vi "DebugProg.vi"() -> ()   [LabVIEW 2012]
uses:
  Instance           5 17Saved   DebugProg .vi
panel:
  out "output array 3":u8[](array[numeric])
  out "VOC Port and states":string[][](array[string])
  out "VOC INPUT PORT states":bool[](array[boolean])
  out "Output Alg Ports":bool[](array[boolean])
  out "Sizes":i32[](array[numeric])
  out "output array 2":u8[](array[numeric])
  out "ALG INPUT PORT states":bool[](array[boolean])
  out "ALG Port and states":string[][](array[string])
  out "Input Alg Ports":bool[](array[boolean])
  out "Output ALG Msg Last Iter":string[][](table)=[["CODE", "PARAM"]]
  out "Output VOC Msg Last Iter":string[][](table)=[["CODE", "PARAM"]]
  out "Curr step ALG msg counter":i32
  out "Curr step VOC MSG counter":i32
  out "Params":string[](array[string])
  in  "STEP SIZE":i32(knob)=1 scale=1.0..10.0
  in  "Mode":bool
  in  "stop 2":bool
  in  "run":bool
  out "Result Input FOR VOC":u8[](array[numeric])
  out "output array":cluster{i32, "Value":string, i32}[](array[cluster])
  in  "Numeric":u8
  in  "Tab Control":T1(tab)=enum."Input VOC Ports "
  out "ALG MSG queue":u8(slide) scale=0.0..5.0
  in  "send msg":bool
  in  "ALG MSG  PARAM":string
  in  "ALG MSG TYPE":string(combo)="0"
  in  "ALG MSG  CODE":string(combo)="1"
  out "VOC MSG queue":u8(slide) scale=0.0..5.0
  in  "send voc msg 2":bool
  in  "VOC MSG  PARAM":string
  in  "VOC MSG TYPE":string(combo)="0"
  in  "VOC MSG  CODE":string(combo)
  in  "New value\n(ALG ports)":i8 min=0
  in  "Controlable\n(ALG ports)":bool
  in  "Set new value\n(ALG ports)":bool
  in  "ALG Input Ports":i32(listbox)
  in  "New value (VOC ports)":i8 min=0
  in  "Controlable (VOC ports)":bool
  in  "Set new value (VOC ports)":bool
  in  "VOC Input Ports":i32(listbox)
  in  "ALG Param type":string(combo)
  in  "ALG Last Interation MSG":i32(listbox)
  out "Alg States":string[][](table)
  out "Output Alg Msg":string[][](table)=[["CODE", "PARAM"]]
  in  "VOC Last Interation MSG":i32(listbox)
  in  "VOC Param type":string(combo)
  out "Output VOC Msg LOG":string[][](table)=[["CODE", "PARAM"]]
  out "VOC States":string[][](table)
  in  "Save as new test":bool
  in  "Save changes in current test":bool
  in  "TEST":string="script_port: 8 /*index*/, 0 /* СЦЕНАРИЙ_ЛОГ_ВХОД_ПИТ_ВЕНТИЛЯТОРА*/ \r\nscript_port: 9 /*index*/, 0 /* СЦЕНАРИЙ_ЛОГ_ВХОД_ПИТ_РЕГ_Т*/ \r\nscript_port: 10 /*index*/, 0 /* СЦЕНАРИЙ_ЛОГ_ВХОД_НАС_ОХЛ*/ \r\nscript_port: 11 /*index*/, 0 /* СЦЕНАРИЙ_ЛОГ_ВХОД_ВАК_НАСОСА*/ \r\nscript_port: 12 /*index*/, 0 /* СЦЕНАРИЙ_ЛОГ_ВХОД_ЗАТВОР_ВАК*/ \r\nscript_port: 13 /*index*/, 0 /* СЦЕНАРИЙ_ЛОГ_ВХОД_САПУН*/ \r\nscript_port: 14 /*index*/, 0 /* СЦЕНАРИЙ_ЛОГ_ВХОД_УСТР_ПЛАВ_ПУСКА*/ \r\nscript_port: 15 /*index*/, 0 /* СЦЕНАРИЙ_ЛОГ_ВХОД_РЕГ_УР*/ \r\nscript_port: 16 /*index*/, 0 /* СЦЕНАРИЙ_ЛОГ_ВХОД_КОМПРЕССОР*/ \r\n\n\n\n\n\n\n\n"
  in  "Tests List":i32(listbox)
  out "voc code":i32[](array[numeric])=[-1, -1, -1, -1, -1, -1, -1, -1, -1, -1, -1, -1, -1, -1, -1, -1, -1, -1, -1, -1, -1, -1, -1, -1, -1, -1, -1, -1, -1, -1, -1, -1, -1, -1, -1, -1, -1, -1, -1, -1, -1, -1, -1, -1, -1, -1, -1, -1, -1, -1, -1, -1, -1, -1, -1, -1, -1, -1, -1, -1, -1, -1, -1, -1, -1, -1, -1, -1, -1, -1, -1, -1, -1, -1, -1, -1, -1, -1, -1, -1, -1, -1, -1, -1, -1, -1, -1, -1, -1, -1, -1, -1, -1, -1, -1, -1, -1, -1, -1, -1, -1, -1, -1, -1, -1, -1, -1, -1, -1, -1, -1, -1, -1, -1, -1, -1, -1, -1, -1, -1, -1, -1, -1, -1, -1, -1, -1, -1, -1, -1, -1, -1, -1, -1, -1, -1, -1, -1, -1, -1, -1, -1, -1, -1, -1, -1, -1, -1, -1, -1, -1, -1, -1, -1, -1, -1, -1, -1, -1, -1, -1, -1, -1, -1, -1, -1, -1, -1, -1, -1, -1, -1, -1, -1, -1, -1, -1, -1, -1, -1, -1, -1, -1, -1, -1, -1, -1, -1, -1, -1, -1, -1, -1, -1, -1, -1, -1, -1, -1, -1, -1, -1, -1, -1, -1, -1, -1, -1, -1, -1, -1, -1, -1, -1, -1, -1, -1, -1, -1, -1, -1, -1, -1, -1, -1, -1, -1, -1, -1, -1, -1, -1, -1, -1, -1, -1, -1, -1, -1, -1, -1, -1, -1, -1, -1, -1, -1, -1, -1, -1]
  out "VOC Out MSG Codes":string[](array[string])=["4", "5", "6", "7", "8", "9", "10", "11", "12", "13", "14", "15", "16", "17", "18", "19", "20", "21", "22", "23", "24", "25", "26", "27", "28", "29", "30", "31", "32", "33"]
  out "VOC Out MSG Names":string[](array[string])=["ПК_ТЕСТ_ГУИ_ОШИБКА_КОДА_КОМАНДЫ_ОТ_ГУИ", "ПК_ТЕСТ_ГУИ_ТЕМПЕРАТУРА_ВОДЫ_В_БАКЕ_ИЗМЕНИЛАСЬ", "ПК_ТЕСТ_ГУИ_ТЕМПЕРАТУРА_ВОДЫ_В_РУБАШКЕ_ИЗМЕНИЛАСЬ", "ПК_ТЕСТ_ГУИ_ТЕМПЕРАТУРА_НАСОСА_ИЗМЕНИЛАСЬ", "ПК_ТЕСТ_ГУИ_ВОДА_В_БАКЕ_ЗАКИПЕЛА", "ПК_ТЕСТ_ГУИ_ВОДА_В_БАКЕ_ЗАМЕРЗЛА", "ПК_ТЕСТ_ГУИ_ТЕМПЕРАТУРА_ВОДЫ_В_БАКЕ_СЛИШКОМ_ВЫСОКАЯ", "ПК_ТЕСТ_ГУИ_ТЕМПЕРАТУРА_ВОДЫ_В_БАКЕ_СЛИШКОМ_НИЗКАЯ", "ПК_ТЕСТ_ГУИ_ТЕМПЕРАТУРА_ОКУЖАЮЩЕЙ_СРЕДЫ_ИЗМЕНИЛАСЬ", "ПК_ТЕСТ_ГУИ_ТЕМПЕРАТУРА_ОКУЖАЮЩЕЙ_СРЕДЫ_СЛИШКОМ_ВЫСОКАЯ", "ПК_ТЕСТ_ГУИ_ТЕМПЕРАТУРА_ОКУЖАЮЩЕЙ_СРЕДЫ_СЛИШКОМ_НИЗКАЯ", "ПК_ТЕСТ_ГУИ_УРОВЕНЬ_ВОДЫ_НОРМ", "ПК_ТЕСТ_ГУИ_УРОВЕНЬ_ВОДЫ_MAX", "ПК_ТЕСТ_ГУИ_УРОВЕНЬ_ВОДЫ_MIN", "ПК_ТЕСТ_ГУИ_ДАВЛЕНИЕ_В_ТРУБЕ_СИДЕРОСТАТА_ИЗМЕНИЛОСЬ", "ПК_ТЕСТ_ГУИ_ДАВЛЕНИЕ_В_ТРУБЕ_СЛИШКОМ_ВЫСОКОЕ", "ПК_ТЕСТ_ГУИ_ДАВЛЕНИЕ_В_ТРУБЕ_СЛИШКОМ_НИЗКОЕ", "ПК_ТЕСТ_ГУИ_ДАВЛЕНИЕ_В_ПАТРУБКЕ_ИЗМЕНИЛОСЬ", "ПК_ТЕСТ_ГУИ_ДАВЛЕНИЕ_В_ПАТРУБКЕ_СЛИШКОМ_ВЫСОКОЕ", "ПК_ТЕСТ_ГУИ_ДАВЛЕНИЕ_В_ПАТРУБКЕ_СЛИШКОМ_НИЗКОЕ", "ПК_ТЕСТ_ГУИ_ДАВЛЕНИЕ_В_БАКЕ_КОМПРЕССОРА_ИЗМЕНИЛОСЬ", "ПК_ТЕСТ_ГУИ_ДАВЛЕНИЕ_В_КОМПРЕССОРЕ_СЛИШКОМ_НИЗКОЕ", "ПК_ТЕСТ_ГУИ_ОШИБКА_ПОПЫТКА_ОТКРЫТЬ_САПУН_ПРИ_ОТКРЫТОМ_ЗАТВОРЕ", "ПК_ТЕСТ_ГУИ_ОШИБКА_ПОПЫТКА_ОТКРЫТЬ_ЗАТВОР_ПРИ_ОТКРЫТОМ_САПУНЕ", "ПК_ТЕСТ_ГУИ_ОШИБКА_ДАВЛЕНИЕ_ПАТРУБКА_ВЫШЕ_ДАВЛЕНИЯ_ТРУБЫ", "ПК_ТЕСТ_ГУИ_ОШИБКА_ВКЛЮЧЕНИЕ_НАГРЕВА_ПРИ_НИЗКОМ_УРОВНЕ_ВОДЫ", "ПК_ТЕСТ_ГУИ_ПОПЫТКА_ЗАПУСКА_УСТР_ПЛАВ_ПУСКА_БЕЗ_ПИТАНИЯ", "ПК_ТЕСТ_ГУИ_ОШИБКА_ВКЛЮЧЕНИЕ_НАСОСА_ОХЛ_ПРИ_НИЗКОМ_УРОВНЕ_ВОДЫ", "ПК_ТЕСТ_ГУИ_ОШИБКА_ПЕРЕГРЕВ_ВАК_НАСОСА", "ПК_ТЕСТ_ГУИ_ОШИБКА_ОТКЛЮЧЕНИЕ_ПИТАНИЯ_ВКН_ПРИ_ЗАПУЩЕННОМ_ВКН"]
  out "output VOC array":cluster{i32, "Value":string, i32}[](array[cluster])=[{-1, "Value"="", 0}, {-1, "Value"="", 0}, {-1, "Value"="", 0}, {-1, "Value"="", 0}, {-1, "Value"="", 0}, {-1, "Value"="", 0}, {-1, "Value"="", 0}, {-1, "Value"="", 0}, {-1, "Value"="", 0}, {-1, "Value"="", 0}, {-1, "Value"="", 0}, {-1, "Value"="", 0}, {-1, "Value"="", 0}, {-1, "Value"="", 0}, {-1, "Value"="", 0}]
  out "input VOC array":cluster{i32, "Value":string, i32}[](array[cluster])
  out "AY states array":cluster{u32, u8}[](array[cluster])
  out "ALG output array":cluster{i32, "Value":string, i32}[](array[cluster])=[{-1, "Value"="", 0}, {-1, "Value"="", 0}, {-1, "Value"="", 0}, {-1, "Value"="", 0}, {-1, "Value"="", 0}]
  out "voc states array":cluster{u32, u8}[](array[cluster])
  out "ALG input array":cluster{i32, "Value":string, i32}[](array[cluster])
  out "VOC_STATES_SET":string[][](array[string])=[["Начало", " ", " ", " ", " ", " "], ["Начало", "НекорректноеСобытие", " ", " ", " ", " "], ["Начало", " ", " ", " ", " ", " "], ["Останов", " ", " ", " ", " ", " "], ["Начало", "Неисправность_вентилятора", " ", " ", " ", " "], ["Включение", "Вентилятор_ВКЛЮЧЕН", " ", " ", " ", " "], ["Выключение", "Вентилятор_ВЫКЛЮЧЕН", " ", " ", " ", " "], ["Начало", "Неисправность_Регулятора_Температуры", " ", " ", " ", " "], ["Включение", "Контроль_температуры_ВКЛЮЧЕН", "Временное_Отключение", "Кипение", " ", " "], ["Включение", "Контроль_температуры_ВЫКЛЮЧЕН", "СамопроизвольноеОхлаждение", "СамопроивольныйНагрев", "Замерзло", "ТепловоеРавновесие"], ["Начало", "Неисправность_регулятора_уровня", " ", " ", " ", " "], ["Включение", "Контроль_Рег_Уровня_ВКЛЮЧЕН", " ", " ", " ", " "], ["Включение", "Контроль_Рег_Уровня_ВЫКЛЮЧЕН", " ", " ", " ", " "], ["Начало", "Неисправность_Насоса_Охлаждения", " ", " ", " ", " "], ["Включение", "Контроль_Насоса_Охлажд_ВКЛЮЧЕН", "НАГРЕВ_НАСОСА_ОХЛАЖД_ВОДЫ", "ОХЛАЖД_НАСОСА_НАГРЕВ_ВОДЫ", "ТепловоеРавновесие", "Авария"], ["Включение", "Контроль_Насоса_Охлажд_ВЫКЛЮЧЕН", "САМОПРОИЗВ_ОХЛАЖД_НАСОСА", "САМОПРОИЗВ_НАГРЕВ_НАСОСА", "ТепловоеРавновесие", " "], ["Начало", "Неисправность_Сапуна", " ", " ", " ", " "], ["Открытие", "Сапун_ОТКРЫТ", " ", " ", " ", " "], ["Выключение", "Сапун_ЗАКРЫТ", " ", " ", " ", " "], ["Начало", "Неисправность_Затвора", " ", " ", " ", " "], ["Открытие", "Затвор_ОТКРЫТ", " ", " ", " ", " "], ["Закрытие", "Затвор_ЗАКРЫТ", " ", " ", " ", " "], ["Начало", "Неисправность_питания_насоса", " ", " ", " ", " "], ["Включение", "Питание_ПОДАНО", " ", " ", " ", " "], ["Выключение", "Задержка_перед_отключением", "Питание_ОТКЛЮЧЕНО", " ", " ", " "], ["Начало", "Неисправность_устр_плав_пуска", " ", " ", " ", " "], ["Включение", "Устр_Плав_Пуска_ЗАПУЩЕНО", "Вакуум", " ", " ", " "], ["Выключение", "Устр_Плав_Пуска_ОСТАНОВЛЕНО", " ", " ", " ", " "], ["Начало", "Исправность_Компрессора", "Неисправность_Компрессора", " ", " ", " "]]
  out "VOC_PROC":string[](array[string])=["Инициализация", "ЧтениеКольцевогоБуфера", "ЗАПОЛНЕНИЕ_ДОСТОВЕРНОСТЕЙ", "АварийноеЗавершениеРаботы", "УПРАВЛЕНИЕ_ВЕНТИЛЯТОРОМ", "ВКЛЮЧЕНИЕ_ВЕНТИЛЯТОРА", "ВЫКЛЮЧЕНИЕ_ВЕНТИЛЯТОРА", "УПРАВЛЕНИЕ_ТЕМПЕРАТУРОЙ", "ВКЛЮЧЕНИЕ_РЕГ_ТЕМПЕРАТУРЫ", "ВЫКЛЮЧЕНИЕ_РЕГ_ТЕМПЕРАТУРЫ", "УПРАВЛЕНИЕ_РЕГУЛЯТОРОМ_УР_ВОДЫ_В_БАКЕ", "ВКЛЮЧЕНИЕ_РЕГ_УРОВНЯ", "ВЫКЛЮЧЕНИЕ_РЕГ_УРОВНЯ", "УПРАВЛЕНИЕ_НАСОСОМ_ОХЛАЖДЕНИЯ", "ВКЛЮЧЕНИЕ_НАСОСА_ОХЛАЖД", "ВЫКЛЮЧЕНИЕ_НАСОСА_ОХЛАЖД", "УПРАВЛЕНИЕ_САПУНОМ", "ОТКРЫТИЕ_САПУНА", "ЗАКРЫТИЕ_САПУНА", "УПРАВЛЕНИЕ_ЗАТВОРОМ", "ОТКРЫТИЕ_ЗАТВОРА", "ЗАКРЫТИЕ_ЗАТВОРА", "УПРАВЛЕНИЕ_ПИТАНИЕМ_ВКН", "ПОДАЧА_ПИТАНИЯ_НА_ВКН", "ОТКЛЮЧЕНИЕ_ПИТАНИЯ_ВКН", "УПРАВЛЕНИЕ_УСТР_ПЛАВ_ПУСКА", "ЗАПУСК_УСТР_ПЛАВ_ПУСКА", "ОСТАНОВ_УСТР_ПЛАВ_ПУСКА", "УПРАВЛЕНИЕ_КОМПРЕССОРОМ"]
  out "Alg Out MSG Codes":string[](array[string])=["0", "1", "2", "3", "4", "5", "6", "7", "8", "9", "10", "11", "12", "13", "14", "15", "16", "41", "42", "43", "44", "45", "46", "47", "48", "49", "50", "51", "52", "53", "54", "55", "56", "57", "58", "59", "60", "61", "62", "63", "64", "65", "66", "67", "68", "69", "70", "71", "72", "73", "74", "75", "76", "77", "78", "79", "80", "81", "82", "83", "84", "85", "86", "87", "88", "89", "90", "91", "92", "93", "94", "95", "96", "97", "98", "99", "100", "101", "102", "103", "104", "105", "106", "107", "108", "109", "110", "111", "112", "113", "114", "115", "116", "117", "118", "119", "120", "121", "122", "123", "124", "125", "126", "127", "128", "129", "130", "135"]
  out "Alg Out MSG Names":string[](array[string])=["ПК_ГУИ_УРОВЕНЬ_ВОДЫ_В_БАКЕ_ОХЛАЖДЕНИЯ_НИЗКИЙ", "ПК_ГУИ_УРОВЕНЬ_ВОДЫ_В_БАКЕ_ОХЛАЖДЕНИЯ_ВЫСОКИЙ", "ПК_ГУИ_УРОВЕНЬ_ВОДЫ_В_БАКЕ_ОХЛАЖДЕНИЯ_В_НОРМЕ", "ПК_ГУИ_ОТКАЗ_ДАТЧИКОВ_УРОВНЯ", "ПК_ГУИ_ТЕМПЕРАТУРА_ВОДЫ_В_БАКЕ_ОХЛАЖДЕНИЯ_НИЗКАЯ", "ПК_ГУИ_ТЕМПЕРАТУРА_ВОДЫ_В_БАКЕ_ОХЛАЖДЕНИЯ_ВЫСОКАЯ", "ПК_ГУИ_ТЕМПЕРАТУРА_ВОДЫ_В_БАКЕ_ОХЛАЖДЕНИЯ_В_НОРМЕ", "ПК_ГУИ_ТЕМПЕРАТУРА_ВОДЫ_В_РУБАШКЕ_ОХЛАЖДЕНИЯ_НИЗКАЯ", "ПК_ГУИ_ТЕМПЕРАТУРА_ВОДЫ_В_РУБАШКЕ_ОХЛАЖДЕНИЯ_ВЫСОКАЯ", "ПК_ГУИ_ТЕМПЕРАТУРА_ВОДЫ_В_РУБАШКЕ_ОХЛАЖДЕНИЯ_В_НОРМЕ", "ПК_ГУИ_ДАВЛЕНИЕ_В_ВАКУУМНОЙ_ТРУБЕ_В_НОРМЕ", "ПК_ГУИ_ДАВЛЕНИЕ_В_ВАКУУМНОЙ_ТРУБЕ_ВНЕ_НОРМЫ", "ПК_ГУИ_СКОРОСТЬ_ОТКАЧКИ_В_НОРМЕ", "ПК_ГУИ_СКОРОСТЬ_ОТКАЧКИ_НИЖЕ_НОРМЫ", "ПК_ГУИ_ДАВЛЕНИЕ_В_БАКЕ_КОМПРЕССОРА_В_НОРМЕ", "ПК_ГУИ_ДАВЛЕНИЕ_В_БАКЕ_КОМПРЕССОРА_ВЫШЕ_НОРМЫ", "ПК_ГУИ_ДАВЛЕНИЕ_В_БАКЕ_КОМПРЕССОРА_НИЖЕ_НОРМЫ", "ПК_ГУИ_ОТКАЗ_ОТКРЫТИЯ_ЗАТВОРА_ВАКУУМНОГО", "ПК_ГУИ_ОТКАЗ_ЗАКРЫТИЯ_ЗАТВОРА_ВАКУУМНОГО", "ПК_ГУИ_ОТКАЗ_ОТКРЫТИЯ_САПУНА", "ПК_ГУИ_ОТКАЗ_ЗАКРЫТИЯ_САПУНА", "ПК_ГУИ_ОТКАЗ_ВКЛЮЧЕНИЯ_ВЕНТИЛЯТОРА", "ПК_ГУИ_ОТКАЗ_ВЫКЛЮЧЕНИЯ_ВЕНТИЛЯТОРА", "ПК_ГУИ_ОТКАЗ_ВКЛЮЧЕНИЯ_УСТР_ПЛАВ_ПУСКА", "ПК_ГУИ_ОТКАЗ_ВЫКЛЮЧЕНИЯ_УСТР_ПЛАВ_ПУСКА", "ПК_ГУИ_ОТКАЗ_ВКЛЮЧЕНИЯ_РЕГУЛЯТОРА_ТЕМПЕРАТУРЫ", "ПК_ГУИ_ОТКАЗ_ВЫКЛЮЧЕНИЯ_РЕГУЛЯТОРА_ТЕМПЕРАТУРЫ", "ПК_ГУИ_ОТКАЗ_ВКЛЮЧЕНИЯ_РЕГУЛЯТОРА_УРОВНЯ", "ПК_ГУИ_ОТКАЗ_ВЫКЛЮЧЕНИЯ_РЕГУЛЯТОРА_УРОВНЯ", "ПК_ГУИ_ОТКАЗ_ВКЛЮЧЕНИЯ_НАСОСА_ОХЛАЖДЕНИЯ", "ПК_ГУИ_ОТКАЗ_ВЫКЛЮЧЕНИЯ_НАСОСА_ОХЛАЖДЕНИЯ", "ПК_ГУИ_ИДЕТ_ВАКУУМИРОВАНИЕ_ОТКАЗ_ВЫПОЛНЕНИЯ_КОМАНДЫ", "ПК_ГУИ_НЕТ_УСЛОВИЙ_ДЛЯ_ВЫПОЛНЕНИЯ_КОМАНДЫ", "ПК_ГУИ_УРОВЕНЬ_ВОДЫ_В_БАКЕ_ОХЛАЖДЕНИЯ_ВНЕ_НОРМЫ_ОТКАЗ_ВЫПОЛНЕНИ", "ПК_ГУИ_ОТРИЦАТЕЛЬНАЯ_ТЕМПЕРАТУРА_ВОДЫ_ОТКАЗ_ВЫПОЛНЕНИЯ_КОМАНДЫ", "ПК_ГУИ_ДАВЛЕНИЕ_В_ПАТРУБКЕ_НЕ_УМЕНЬШАЕТСЯ", "ПК_ГУИ_ДАВЛЕНИЕ_В_ВАК_ТРУБЕ_НЕ_УМЕНЬШАЕТСЯ", "ПК_ГУИ_ВАКУУМИРОВАНИЕ_УСПЕШНО_ЗАВЕРШЕНО", "ПК_ГУИ_ОТКАЗ_ВКЛЮЧЕНИЯ_ПИТАНИЯ_ВАКУУМНОГО_НАСОСА", "ПК_ГУИ_ОТКАЗ_ВЫКЛЮЧЕНИЯ_ПИТАНИЯ_ВАКУУМНОГО_НАСОСА", "ПК_ГУИ_АВАРИЯ_НЕДОСТОВЕРНЫЕ_ДАННЫЕ_ОБОРУДОВАНИЯ_ВАК_СИСТЕМЫ", "ПК_ГУИ_ВЕНТИЛЯТОР_ВКЛЮЧЕН", "ПК_ГУИ_ВЕНТИЛЯТОР_ВЫКЛЮЧЕН", "ПК_ГУИ_СПОНТАННОЕ_ВЫКЛЮЧЕНИЕ_ВЕНТИЛЯТОРА", "ПК_ГУИ_СПОНТАННОЕ_ВКЛЮЧЕНИЕ_ВЕНТИЛЯТОРА", "ПК_ГУИ_ЗАТВОР_ВАКУУМНЫЙ_ОТКРЫТ", "ПК_ГУИ_ЗАТВОР_ВАКУУМНЫЙ_ЗАКРЫТ", "ПК_ГУИ_СРЕДНЕЕ_СОСТОЯНИЕ_ЗАТВОРА_ВАКУУМНОГО", "ПК_ГУИ_СОСТОЯНИЕ_ОШИБКИ_ЗАТВОРА_ВАКУУМНОГО", "ПК_ГУИ_СПОНТАННОЕ_ОТКРЫТИЕ_ЗАТ_ВАКУУМНОГО", "ПК_ГУИ_СПОНТАННОЕ_ЗАКРЫТИЕ_ЗАТ_ВАКУУМНОГО", "ПК_ГУИ_САПУН_ОТКРЫТ", "ПК_ГУИ_САПУН_ЗАКРЫТ", "ПК_ГУИ_СПОНТАННОЕ_ОТКРЫТИЕ_САПУНА", "ПК_ГУИ_СПОНТАННОЕ_ЗАКРЫТИЕ_САПУНА", "ПК_ГУИ_ПИТАНИЕ_ВАКУУМНОГО_НАСОСА_ВКЛЮЧЕНО", "ПК_ГУИ_ПИТАНИЕ_ВАКУУМНОГО_НАСОСА_ВЫКЛЮЧЕНО", "ПК_ГУИ_СПОНТАННОЕ_ВКЛЮЧЕНИЕ_ВАКУУМНОГО_НАСОСА", "ПК_ГУИ_СПОНТАННОЕ_ВЫКЛЮЧЕНИЕ_ВАКУУМНОГО_НАСОСА", "ПК_ГУИ_ПИТАНИЕ_РЕГУЛЯТОРА_ТЕМПЕРАТУРЫ_ВКЛЮЧЕНО", "ПК_ГУИ_ПИТАНИЕ_РЕГУЛЯТОРА_ТЕМПЕРАТУРЫ_ВЫКЛЮЧЕНО", "ПК_ГУИ_СПОНТАННОЕ_ВКЛЮЧЕНИЕ_РЕГУЛЯТОРА_ТЕМПЕРАТУРЫ", "ПК_ГУИ_СПОНТАННОЕ_ВЫКЛЮЧЕНИЕ_РЕГУЛЯТОРА_ТЕМПЕРАТУРЫ", "ПК_ГУИ_ПИТАНИЕ_РЕГУЛЯТОРА_УРОВНЯ_ВКЛЮЧЕНО", "ПК_ГУИ_ПИТАНИЕ_РЕГУЛЯТОРА_УРОВНЯ_ВЫКЛЮЧЕНО", "ПК_ГУИ_СПОНТАННОЕ_ВКЛЮЧЕНИЕ_РЕГУЛЯТОРА_УРОВНЯ", "ПК_ГУИ_СПОНТАННОЕ_ВЫКЛЮЧЕНИЕ_РЕГУЛЯТОРА_УРОВНЯ", "ПК_ГУИ_ПИТАНИЕ_НАСОСА_ОХЛАЖДЕНИЯ_ВКЛЮЧЕНО", "ПК_ГУИ_ПИТАНИЕ_НАСОСА_ОХЛАЖДЕНИЯ_ВЫКЛЮЧЕНО", "ПК_ГУИ_СПОНТАННОЕ_ВКЛЮЧЕНИЕ_НАСОСА_ОХЛАЖДЕНИЯ", "ПК_ГУИ_СПОНТАННОЕ_ВЫКЛЮЧЕНИЕ_НАСОСА_ОХЛАЖДЕНИЯ", "ПК_ГУИ_УСТРОЙСТВО_ПЛАВНОГО_ПУСКА_ВКЛЮЧЕНО", "ПК_ГУИ_УСТРОЙСТВО_ПЛАВНОГО_ПУСКА_ВЫКЛЮЧЕНО", "ПК_ГУИ_СПОНТАННОЕ_ВКЛЮЧЕНИЕ_УСТРОЙСТВА_ПЛАВНОГО_ПУСКА", "ПК_ГУИ_СПОНТАННОЕ_ВЫКЛЮЧЕНИЕ_УСТРОЙСТВА_ПЛАВНОГО_ПУСКА", "ПК_ГУИ_ОТКАЗ_ВАКУУМИРОВАНИЯ", "ПК_ГУИ_ОТКАЗ_ВКЛЮЧЕНИЯ_ВАКУУМНОЙ_ПОДСИСТЕМЫ", "ПК_ГУИ_ОТКАЗ_ВЫКЛЮЧЕНИЯ_ВАКУУМНОЙ_ПОДСИСТЕМЫ", "ПК_ГУИ_ЕСТЬ_ДОСТОВЕРНОСТЬ_КОНТРОЛЯ_ОТКРЫТИЯ_ЗАТВОРА_ВАКУУМНОГО", "ПК_ГУИ_НЕТ_ДОСТОВЕРНОСТИ_КОНТРОЛЯ_ОТКРЫТИЯ_ЗАТВОРА_ВАКУУМНОГО", "ПК_ГУИ_ЕСТЬ_ДОСТОВЕРНОСТЬ_КОНТРОЛЯ_ЗАКРЫТИЯ_ЗАТВОРА_ВАКУУМНОГО", "ПК_ГУИ_НЕТ_ДОСТОВЕРНОСТИ_КОНТРОЛЯ_ЗАКРЫТИЯ_ЗАТВОРА_ВАКУУМНОГО", "ПК_ГУИ_ЕСТЬ_ДОСТОВЕРНОСТЬ_КОНТРОЛЯ_САПУНА", "ПК_ГУИ_НЕТ_ДОСТОВЕРНОСТИ_КОНТРОЛЯ_САПУНА", "ПК_ГУИ_ЕСТЬ_ДОСТОВЕРНОСТЬ_КОНТРОЛЯ_УСТР_ПЛАВ_ПУСКА", "ПК_ГУИ_НЕТ_ДОСТОВЕРНОСТИ_КОНТРОЛЯ_УСТР_ПЛАВ_ПУСКА", "ПК_ГУИ_ЕСТЬ_ДОСТОВЕРНОСТЬ_КОНТРОЛЯ_ПИТ_ВАК_НАСОСА", "ПК_ГУИ_НЕТ_ДОСТОВЕРНОСТИ_КОНТРОЛЯ_ПИТ_ВАК_НАСОСА", "ПК_ГУИ_ЕСТЬ_ДОСТОВЕРНОСТЬ_КОНТРОЛЯ_ПИТ_ВЕНТИЛЯТОРА", "ПК_ГУИ_НЕТ_ДОСТОВЕРНОСТИ_КОНТРОЛЯ_ПИТ_ВЕНТИЛЯТОРА", "ПК_ГУИ_ЕСТЬ_ДОСТОВЕРНОСТЬ_РЕГ_ТЕМПЕРАТУРЫ", "ПК_ГУИ_НЕТ_ДОСТОВЕРНОСТИ_КОНТРОЛЯ_ПИТ_РЕГ_ТЕМПЕРАТУРЫ", "ПК_ГУИ_ЕСТЬ_ДОСТОВЕРНОСТЬ_РЕГ_УРОВНЯ", "ПК_ГУИ_НЕТ_ДОСТОВЕРНОСТИ_КОНТРОЛЯ_ПИТ_РЕГ_УРОВНЯ", "ПК_ГУИ_ЕСТЬ_ДОСТОВЕРНОСТЬ_МИНИМ_УР_ВОДЫ", "ПК_ГУИ_НЕТ_ДОСТОВЕРНОСТИ_МИНИМ_УР_ВОДЫ", "ПК_ГУИ_ЕСТЬ_ДОСТОВЕРНОСТЬ_МАКСИМ_УР_ВОДЫ", "ПК_ГУИ_НЕТ_ДОСТОВЕРНОСТИ_МАКСИМ_УР_ВОДЫ", "ПК_ГУИ_ЕСТЬ_ДОСТОВЕРНОСТЬ_КОНТРОЛЯ_ПИТ_НАСОСА_ОХЛ", "ПК_ГУИ_НЕТ_ДОСТОВЕРНОСТИ_КОНТРОЛЯ_ПИТ_НАСОСА_ОХЛ", "ПК_ГУИ_ВАКУУМИРОВАНИЕ_ТРУБЫ_ВКЛЮЧЕНО", "ПК_ГУИ_ВАКУУМИРОВАНИЕ_ТРУБЫ_ВЫКЛЮЧЕНО", "ПК_ГУИ_ФП_P_ВбакеКомпрессора", "ПК_ГУИ_ФП_P_Впатрубке", "ПК_ГУИ_ФП_T_Врубашке", "ПК_ГУИ_ФП_T_Вбаке", "ПК_ГУИ_ФП_P_ВтрубеСидер", "ПК_ГУИ_ОШИБКА_КОДА_КОМАНДЫ_ОТ_ГУИ"]
  out "AY_STATES_SET":string[][](array[string])=[["Начало", "ВосстановлениеУправления", "НачалоРаботы", " ", " ", " ", " ", " ", " ", " ", " ", " ", " ", " ", " ", " ", " ", " ", " ", " ", " ", " ", " ", " ", " ", " ", " ", " ", " ", " "], ["Начало", " ", " ", " ", " ", " ", " ", " ", " ", " ", " ", " ", " ", " ", " ", " ", " ", " ", " ", " ", " ", " ", " ", " ", " ", " ", " ", " ", " ", " "], ["Начало", "ОстановПроцессов", "СообК_ГУИ_НЕТ_ДОСТОВЕРНОСТИ", "НарушениеСвязи", " ", " ", " ", " ", " ", " ", " ", " ", " ", " ", " ", " ", " ", " ", " ", " ", " ", " ", " ", " ", " ", " ", " ", " ", " ", " "], ["Начало", "СменаСостоянияВКЛ", "СменаСостоянияВЫКЛ", "ТрафикПауза", "НарушениеСвязи", " ", " ", " ", " ", " ", " ", " ", " ", " ", " ", " ", " ", " ", " ", " ", " ", " ", " ", " ", " ", " ", " ", " ", " ", " "], ["Начало", "СообК_ГУИ_ЕСТЬ_ДОСТОВЕРНОСТЬ", "ОжиданиеНедостоверности", "СообК_ГУИ_НЕТ_ДОСТОВЕРНОСТИ", "ОжиданиеЕстьДостоверность", "НарушениеСвязи", " ", " ", " ", " ", " ", " ", " ", " ", " ", " ", " ", " ", " ", " ", " ", " ", " ", " ", " ", " ", " ", " ", " ", " "], ["Начало", "СообК_ГУИ_ЕСТЬ_ДОСТОВЕРНОСТЬ", "ОжиданиеНедостоверности", "СообК_ГУИ_НЕТ_ДОСТОВЕРНОСТИ", "ОжиданиеЕстьДостоверность", "НарушениеСвязи", " ", " ", " ", " ", " ", " ", " ", " ", " ", " ", " ", " ", " ", " ", " ", " ", " ", " ", " ", " ", " ", " ", " ", " "], ["Начало", "СообК_ГУИ_ЕСТЬ_ДОСТОВЕРНОСТЬ", "ОжиданиеНедостоверности", "СообК_ГУИ_НЕТ_ДОСТОВЕРНОСТИ", "ОжиданиеЕстьДостоверность", "НарушениеСвязи", " ", " ", " ", " ", " ", " ", " ", " ", " ", " ", " ", " ", " ", " ", " ", " ", " ", " ", " ", " ", " ", " ", " ", " "], ["Начало", "СообК_ГУИ_ЕСТЬ_ДОСТОВЕРНОСТЬ", "ОжиданиеНедостоверности", "СообК_ГУИ_НЕТ_ДОСТОВЕРНОСТИ", "ОжиданиеЕстьДостоверность", "НарушениеСвязи", " ", " ", " ", " ", " ", " ", " ", " ", " ", " ", " ", " ", " ", " ", " ", " ", " ", " ", " ", " ", " ", " ", " ", " "], ["Начало", "СообК_ГУИ_ЕСТЬ_ДОСТОВЕРНОСТЬ", "ОжиданиеНедостоверности", "СообК_ГУИ_НЕТ_ДОСТОВЕРНОСТИ", "ОжиданиеЕстьДостоверность", "НарушениеСвязи", " ", " ", " ", " ", " ", " ", " ", " ", " ", " ", " ", " ", " ", " ", " ", " ", " ", " ", " ", " ", " ", " ", " ", " "], ["Начало", "СообК_ГУИ_ЕСТЬ_ДОСТОВЕРНОСТЬ", "ОжиданиеНедостоверности", "СообК_ГУИ_НЕТ_ДОСТОВЕРНОСТИ", "ОжиданиеЕстьДостоверность", "НарушениеСвязи", " ", " ", " ", " ", " ", " ", " ", " ", " ", " ", " ", " ", " ", " ", " ", " ", " ", " ", " ", " ", " ", " ", " ", " "], ["Начало", "СообК_ГУИ_ЕСТЬ_ДОСТОВЕРНОСТЬ", "ОжиданиеНедостоверности", "СообК_ГУИ_НЕТ_ДОСТОВЕРНОСТИ", "ОжиданиеЕстьДостоверность", "НарушениеСвязи", " ", " ", " ", " ", " ", " ", " ", " ", " ", " ", " ", " ", " ", " ", " ", " ", " ", " ", " ", " ", " ", " ", " ", " "], ["Начало", "СообК_ГУИ_ЕСТЬ_ДОСТОВЕРНОСТЬ", "ОжиданиеНедостоверности", "СообК_ГУИ_НЕТ_ДОСТОВЕРНОСТИ", "ОжиданиеЕстьДостоверность", "НарушениеСвязи", " ", " ", " ", " ", " ", " ", " ", " ", " ", " ", " ", " ", " ", " ", " ", " ", " ", " ", " ", " ", " ", " ", " ", " "], ["Начало", "СообК_ГУИ_ЕСТЬ_ДОСТОВЕРНОСТЬ", "ОжиданиеНедостоверности", "СообК_ГУИ_НЕТ_ДОСТОВЕРНОСТИ", "ОжиданиеЕстьДостоверность", "НарушениеСвязи", " ", " ", " ", " ", " ", " ", " ", " ", " ", " ", " ", " ", " ", " ", " ", " ", " ", " ", " ", " ", " ", " ", " ", " "], ["Начало", "СообК_ГУИ_ЕСТЬ_ДОСТОВЕРНОСТЬ", "ОжиданиеНедостоверности", "СообК_ГУИ_НЕТ_ДОСТОВЕРНОСТИ", "ОжиданиеЕстьДостоверность", "НарушениеСвязи", " ", " ", " ", " ", " ", " ", " ", " ", " ", " ", " ", " ", " ", " ", " ", " ", " ", " ", " ", " ", " ", " ", " ", " "], ["Начало", "СообК_ГУИ_ЕСТЬ_ДОСТОВЕРНОСТЬ", "ОжиданиеНедостоверности", "СообК_ГУИ_НЕТ_ДОСТОВЕРНОСТИ", "ОжиданиеЕстьДостоверность", "НарушениеСвязи", " ", " ", " ", " ", " ", " ", " ", " ", " ", " ", " ", " ", " ", " ", " ", " ", " ", " ", " ", " ", " ", " ", " ", " "], ["Начало", " ", " ", " ", " ", " ", " ", " ", " ", " ", " ", " ", " ", " ", " ", " ", " ", " ", " ", " ", " ", " ", " ", " ", " ", " ", " ", " ", " ", " "], ["Начало", " ", " ", " ", " ", " ", " ", " ", " ", " ", " ", " ", " ", " ", " ", " ", " ", " ", " ", " ", " ", " ", " ", " ", " ", " ", " ", " ", " ", " "], ["Начало", "КонтрольВыполненияК", "КонтрольИзмененияНП", "НекорректноеСобытие", "НарушениеСвязи", " ", " ", " ", " ", " ", " ", " ", " ", " ", " ", " ", " ", " ", " ", " ", " ", " ", " ", " ", " ", " ", " ", " ", " ", " "], ["Анализ", "ПодтверждениеИзмененияНП", "НекорректноеСобытие", "НарушениеСвязи", " ", " ", " ", " ", " ", " ", " ", " ", " ", " ", " ", " ", " ", " ", " ", " ", " ", " ", " ", " ", " ", " ", " ", " ", " ", " "], ["Анализ", "НекорректноеСобытие", "ПередачаСообщенияСПараметромГУИ", "НарушениеСвязи", " ", " ", " ", " ", " ", " ", " ", " ", " ", " ", " ", " ", " ", " ", " ", " ", " ", " ", " ", " ", " ", " ", " ", " ", " ", " "], ["Начало", "КонтрольИзменения", "СообщОбИзменении", "ТрафикПауза", "НарушениеСвязи", " ", " ", " ", " ", " ", " ", " ", " ", " ", " ", " ", " ", " ", " ", " ", " ", " ", " ", " ", " ", " ", " ", " ", " ", " "], ["Начало", "КонтрольИзменения", "СообщОбИзменении", "ТрафикПауза", "НарушениеСвязи", " ", " ", " ", " ", " ", " ", " ", " ", " ", " ", " ", " ", " ", " ", " ", " ", " ", " ", " ", " ", " ", " ", " ", " ", " "], ["Начало", "КонтрольИзменения", "СообщОбИзменении", "ТрафикПауза", "НарушениеСвязи", " ", " ", " ", " ", " ", " ", " ", " ", " ", " ", " ", " ", " ", " ", " ", " ", " ", " ", " ", " ", " ", " ", " ", " ", " "], ["Начало", "КонтрольИзменения", "СообщОбИзменении", "ТрафикПауза", "НарушениеСвязи", " ", " ", " ", " ", " ", " ", " ", " ", " ", " ", " ", " ", " ", " ", " ", " ", " ", " ", " ", " ", " ", " ", " ", " ", " "], ["Начало", "КонтрольИзменения", "СообщОбИзменении", "ТрафикПауза", "НарушениеСвязи", " ", " ", " ", " ", " ", " ", " ", " ", " ", " ", " ", " ", " ", " ", " ", " ", " ", " ", " ", " ", " ", " ", " ", " ", " "], ["Начало", "АнализОткачки", " ", " ", " ", " ", " ", " ", " ", " ", " ", " ", " ", " ", " ", " ", " ", " ", " ", " ", " ", " ", " ", " ", " ", " ", " ", " ", " ", " "], ["Начало", "ДавлениеНормальное", "ДавлениеВысокое", "Задержка", "НарушениеСвязи", " ", " ", " ", " ", " ", " ", " ", " ", " ", " ", " ", " ", " ", " ", " ", " ", " ", " ", " ", " ", " ", " ", " ", " ", " "], ["Начало", "НизкийУровеньВоды", "ВысокийУровеньВоды", "УровеньВодыВнорме", "Задержка", "НарушениеСвязи", " ", " ", " ", " ", " ", " ", " ", " ", " ", " ", " ", " ", " ", " ", " ", " ", " ", " ", " ", " ", " ", " ", " ", " "], ["Начало", "НизкаяТемператураВоды", "ВысокаяТемператураВоды", "ТемператураВнорме", "Задержка", "НарушениеСвязи", " ", " ", " ", " ", " ", " ", " ", " ", " ", " ", " ", " ", " ", " ", " ", " ", " ", " ", " ", " ", " ", " ", " ", " "], ["Начало", "НизкаяТемператураВоды", "ВысокаяТемператураВоды", "ТемператураВнорме", "Задержка", "НарушениеСвязи", " ", " ", " ", " ", " ", " ", " ", " ", " ", " ", " ", " ", " ", " ", " ", " ", " ", " ", " ", " ", " ", " ", " ", " "], ["Начало", "НизкоеДавление", "ДавлениеВнорме", "Задержка", "НарушениеСвязи", " ", " ", " ", " ", " ", " ", " ", " ", " ", " ", " ", " ", " ", " ", " ", " ", " ", " ", " ", " ", " ", " ", " ", " ", " "], ["Начало", "КонтрольВключения", "ПередачаСообщения", "Ошибка", "НарушениеСвязи", " ", " ", " ", " ", " ", " ", " ", " ", " ", " ", " ", " ", " ", " ", " ", " ", " ", " ", " ", " ", " ", " ", " ", " ", " "], ["Начало", "КонтрольВыключения", "ПередачаСообщения", "Ошибка", "НарушениеСвязи", " ", " ", " ", " ", " ", " ", " ", " ", " ", " ", " ", " ", " ", " ", " ", " ", " ", " ", " ", " ", " ", " ", " ", " ", " "], ["Начало", "СменаСостоянияВКЛ", "СменаСостоянияВЫКЛ", "НарушениеСвязи", " ", " ", " ", " ", " ", " ", " ", " ", " ", " ", " ", " ", " ", " ", " ", " ", " ", " ", " ", " ", " ", " ", " ", " ", " ", " "], ["Контроль", "Ошибка", "НарушениеСвязи", " ", " ", " ", " ", " ", " ", " ", " ", " ", " ", " ", " ", " ", " ", " ", " ", " ", " ", " ", " ", " ", " ", " ", " ", " ", " ", " "], ["Контроль", "Ошибка", "НарушениеСвязи", " ", " ", " ", " ", " ", " ", " ", " ", " ", " ", " ", " ", " ", " ", " ", " ", " ", " ", " ", " ", " ", " ", " ", " ", " ", " ", " "], ["Начало", "СменаСостоянияСреднего", "СменаСостоянияЗакрытия", "СменаСостоянияОткрытия", "СменаСостоянияОшибки", "НарушениеСвязи", " ", " ", " ", " ", " ", " ", " ", " ", " ", " ", " ", " ", " ", " ", " ", " ", " ", " ", " ", " ", " ", " ", " ", " "], ["Начало", "Контроль", "ПередачаСообщения", "Ошибка", "НарушениеСвязи", " ", " ", " ", " ", " ", " ", " ", " ", " ", " ", " ", " ", " ", " ", " ", " ", " ", " ", " ", " ", " ", " ", " ", " ", " "], ["Начало", "Контроль", "ПередачаСообщения", "Ошибка", "НарушениеСвязи", " ", " ", " ", " ", " ", " ", " ", " ", " ", " ", " ", " ", " ", " ", " ", " ", " ", " ", " ", " ", " ", " ", " ", " ", " "], ["КонтрольЗакрытия", "Ошибка", "НарушениеСвязи", " ", " ", " ", " ", " ", " ", " ", " ", " ", " ", " ", " ", " ", " ", " ", " ", " ", " ", " ", " ", " ", " ", " ", " ", " ", " ", " "], ["Контроль", "Ошибка", "НарушениеСвязи", " ", " ", " ", " ", " ", " ", " ", " ", " ", " ", " ", " ", " ", " ", " ", " ", " ", " ", " ", " ", " ", " ", " ", " ", " ", " ", " "], ["Начало", "КонтрольОткрытия", "ПередачаСообщения", "Ошибка", "НарушениеСвязи", " ", " ", " ", " ", " ", " ", " ", " ", " ", " ", " ", " ", " ", " ", " ", " ", " ", " ", " ", " ", " ", " ", " ", " ", " "], ["Начало", "КонтрольЗакрытия", "ПередачаСообщения", "Ошибка", "НарушениеСвязи", " ", " ", " ", " ", " ", " ", " ", " ", " ", " ", " ", " ", " ", " ", " ", " ", " ", " ", " ", " ", " ", " ", " ", " ", " "], ["Начало", "СменаСостоянияВКЛ", "СменаСостоянияВЫКЛ", "НарушениеСвязи", " ", " ", " ", " ", " ", " ", " ", " ", " ", " ", " ", " ", " ", " ", " ", " ", " ", " ", " ", " ", " ", " ", " ", " ", " ", " "], ["КонтрольЗакрытия", "Ошибка", "НарушениеСвязи", " ", " ", " ", " ", " ", " ", " ", " ", " ", " ", " ", " ", " ", " ", " ", " ", " ", " ", " ", " ", " ", " ", " ", " ", " ", " ", " "], ["Контроль", "Ошибка", "НарушениеСвязи", " ", " ", " ", " ", " ", " ", " ", " ", " ", " ", " ", " ", " ", " ", " ", " ", " ", " ", " ", " ", " ", " ", " ", " ", " ", " ", " "], ["Начало", "КонтрольВключения", "ПередачаСообщения", "Ошибка", "НарушениеСвязи", " ", " ", " ", " ", " ", " ", " ", " ", " ", " ", " ", " ", " ", " ", " ", " ", " ", " ", " ", " ", " ", " ", " ", " ", " "], ["Начало", "КонтрольВыключения", "Ошибка", "НарушениеСвязи", "ПередачаСообщения", " ", " ", " ", " ", " ", " ", " ", " ", " ", " ", " ", " ", " ", " ", " ", " ", " ", " ", " ", " ", " ", " ", " ", " ", " "], ["Начало", "СменаСостоянияВКЛ", "СменаСостоянияВЫКЛ", "НарушениеСвязи", " ", " ", " ", " ", " ", " ", " ", " ", " ", " ", " ", " ", " ", " ", " ", " ", " ", " ", " ", " ", " ", " ", " ", " ", " ", " "], ["Контроль", "Ошибка", "НарушениеСвязи", " ", " ", " ", " ", " ", " ", " ", " ", " ", " ", " ", " ", " ", " ", " ", " ", " ", " ", " ", " ", " ", " ", " ", " ", " ", " ", " "], ["Контроль", "Ошибка", "НарушениеСвязи", " ", " ", " ", " ", " ", " ", " ", " ", " ", " ", " ", " ", " ", " ", " ", " ", " ", " ", " ", " ", " ", " ", " ", " ", " ", " ", " "], ["Начало", "КонтрольВключения", "ПередачаСообщения", "Ошибка", "НарушениеСвязи", " ", " ", " ", " ", " ", " ", " ", " ", " ", " ", " ", " ", " ", " ", " ", " ", " ", " ", " ", " ", " ", " ", " ", " ", " "], ["Начало", "КонтрольВыключения", "ПередачаСообщения", "Ошибка", "НарушениеСвязи", " ", " ", " ", " ", " ", " ", " ", " ", " ", " ", " ", " ", " ", " ", " ", " ", " ", " ", " ", " ", " ", " ", " ", " ", " "], ["Начало", "СменаСостоянияВКЛ", "СменаСостоянияВЫКЛ", "НарушениеСвязи", " ", " ", " ", " ", " ", " ", " ", " ", " ", " ", " ", " ", " ", " ", " ", " ", " ", " ", " ", " ", " ", " ", " ", " ", " ", " "], ["Контроль", "Ошибка", "НарушениеСвязи", " ", " ", " ", " ", " ", " ", " ", " ", " ", " ", " ", " ", " ", " ", " ", " ", " ", " ", " ", " ", " ", " ", " ", " ", " ", " ", " "], ["Контроль", "Ошибка", "НарушениеСвязи", " ", " ", " ", " ", " ", " ", " ", " ", " ", " ", " ", " ", " ", " ", " ", " ", " ", " ", " ", " ", " ", " ", " ", " ", " ", " ", " "], ["Начало", "Контроль", "ПередачаСообщения", "Ошибка", "НарушениеСвязи", " ", " ", " ", " ", " ", " ", " ", " ", " ", " ", " ", " ", " ", " ", " ", " ", " ", " ", " ", " ", " ", " ", " ", " ", " "], ["Начало", "Контроль", "ПередачаСообщения", "Ошибка", "НарушениеСвязи", " ", " ", " ", " ", " ", " ", " ", " ", " ", " ", " ", " ", " ", " ", " ", " ", " ", " ", " ", " ", " ", " ", " ", " ", " "], ["Начало", "СменаСостоянияВКЛ", "СменаСостоянияВЫКЛ", "НарушениеСвязи", " ", " ", " ", " ", " ", " ", " ", " ", " ", " ", " ", " ", " ", " ", " ", " ", " ", " ", " ", " ", " ", " ", " ", " ", " ", " "], ["Контроль", "Ошибка", "НарушениеСвязи", " ", " ", " ", " ", " ", " ", " ", " ", " ", " ", " ", " ", " ", " ", " ", " ", " ", " ", " ", " ", " ", " ", " ", " ", " ", " ", " "], ["Контроль", "Ошибка", "НарушениеСвязи", " ", " ", " ", " ", " ", " ", " ", " ", " ", " ", " ", " ", " ", " ", " ", " ", " ", " ", " ", " ", " ", " ", " ", " ", " ", " ", " "], ["Начало", "ВключениеПитания", "Контроль", "ПередачаСообщения", "Ошибка", "НарушениеСвязи", " ", " ", " ", " ", " ", " ", " ", " ", " ", " ", " ", " ", " ", " ", " ", " ", " ", " ", " ", " ", " ", " ", " ", " "], ["Начало", "Контроль", "ПередачаСообщения", "Ошибка", "НарушениеСвязи", " ", " ", " ", " ", " ", " ", " ", " ", " ", " ", " ", " ", " ", " ", " ", " ", " ", " ", " ", " ", " ", " ", " ", " ", " "], ["Начало", "СменаСостоянияВКЛ", "СменаСостоянияВЫКЛ", "НарушениеСвязи", " ", " ", " ", " ", " ", " ", " ", " ", " ", " ", " ", " ", " ", " ", " ", " ", " ", " ", " ", " ", " ", " ", " ", " ", " ", " "], ["Контроль", "Ошибка", "НарушениеСвязи", " ", " ", " ", " ", " ", " ", " ", " ", " ", " ", " ", " ", " ", " ", " ", " ", " ", " ", " ", " ", " ", " ", " ", " ", " ", " ", " "], ["Контроль", "Ошибка", "НарушениеСвязи", " ", " ", " ", " ", " ", " ", " ", " ", " ", " ", " ", " ", " ", " ", " ", " ", " ", " ", " ", " ", " ", " ", " ", " ", " ", " ", " "], ["Начало", "Контроль", "ПередачаСообщения", "Ошибка", "НарушениеСвязи", " ", " ", " ", " ", " ", " ", " ", " ", " ", " ", " ", " ", " ", " ", " ", " ", " ", " ", " ", " ", " ", " ", " ", " ", " "], ["Начало", "КонтрольВыключения", "ПередачаСообщения", "Ошибка", "НарушениеСвязи", " ", " ", " ", " ", " ", " ", " ", " ", " ", " ", " ", " ", " ", " ", " ", " ", " ", " ", " ", " ", " ", " ", " ", " ", " "], ["Начало", "СменаСостоянияВКЛ", "СменаСостоянияВЫКЛ", "НарушениеСвязи", " ", " ", " ", " ", " ", " ", " ", " ", " ", " ", " ", " ", " ", " ", " ", " ", " ", " ", " ", " ", " ", " ", " ", " ", " ", " "], ["Контроль", "Ошибка", "НарушениеСвязи", " ", " ", " ", " ", " ", " ", " ", " ", " ", " ", " ", " ", " ", " ", " ", " ", " ", " ", " ", " ", " ", " ", " ", " ", " ", " ", " "], ["Контроль", "Ошибка", "НарушениеСвязи", " ", " ", " ", " ", " ", " ", " ", " ", " ", " ", " ", " ", " ", " ", " ", " ", " ", " ", " ", " ", " ", " ", " ", " ", " ", " ", " "], ["Начало", "ПроверкаНеобходимостиВакуумирования", "ПередачаСообщения", "КонтрольВключенияВакПодсистемы", "ЗапоминаемДавлениеВвакуумнойТрубе", "КонтрольТемпературыРубашки", "КонтрольРаботыОборудования", "КонтрольДавления", "СообщениеОКонцеВакуумирования", "ПаузаНаРазвакуумированиеТрубы", "ПаузаНаОткачкуВвакуумнойТрубе", "ПроверкаУменьшенияДавленияВпатрубке", "ОткачкаОтсутствует", "ВыключениеВакуумнойПодсистемы", "СообщениеОбОтказеВакуумирования", "НарушениеСвязи", " ", " ", " ", " ", " ", " ", " ", " ", " ", " ", " ", " ", " ", " "], ["Начало", "ПередачаСообщения", "ВыключениеВакуумнойПодсистемы", "НарушениеСвязи", " ", " ", " ", " ", " ", " ", " ", " ", " ", " ", " ", " ", " ", " ", " ", " ", " ", " ", " ", " ", " ", " ", " ", " ", " ", " "], ["Начало", "ВключениеПитанияРегУровня", "КонтрольВключенияПитРегУр", "КонтрольГотовностиУровняВодыБО", "ВключениеРегТ", "КонтрольВключенияРегТ", "КонтрольПревышенияТемпературыВодыБО", "КонтрольГотовностиТемпературыВодыБО", "ВключаемВентилятор", "КонтрольВключенияВентилятора", "КонтрольВключенияПитанияНасосаОхлаждения", "КонтрольЗакрытияЗатвораВакуумного", "КонтрольОткрытияСапуна", "КонтрольТемпературыРубашки", "ПодачаПитанияНаВакуумныйНасос", "КонтрольПитанияВакуумногоНасоса", "ВключениеУстройстваПлавногоПуска", "КонтрольВлюченияПлавногоПуска", "ТаймаутПередЗакрытиемСапуна", "ЗакрытиеСапуна", "КонтрольЗакрытияСапуна", "ЗапоминаемДавлениеВпатрубке", "КонтрольДавления", "ПаузаНаОткачкуВпатрубке", "ПроверкаУменьшенияДавленияВпатрубке", "КонтрольОткрытияЗВ", "Ошибка", "ВыключениеПоОшибке", "СообщениеОбОтказеВакуумирования", "НарушениеСвязи"], ["Начало", "КонтрольЗакрытияЗатвораВакуумного", "КонтрольОткрытияСапуна", "ТаймаутПередВыключениемПитанияВакуумногоНасоса", "ВыключаемУППВакуумногоНасоса", "КонтрольВыключенияПитанияУППВакуумногоНасоса", "КонтрольВыключенияПитанияВакуумногоНасоса", "КонтрольВыключенияНасосаОхлаждения", "КонтрольВыключенияВентилятора", "СообщениеОбОтказеВыклВакСистемы", "НарушениеСвязи", " ", " ", " ", " ", " ", " ", " ", " ", " ", " ", " ", " ", " ", " ", " ", " ", " ", " ", " "]]
  out "AY_PROC":string[](array[string])=["Инициализация", "ОстановВсехПроцессовИстартПроцИнициализация", "КонтрольДостоверности", "КонтрольДостоверностиОткрытияЗатвораВакуумного", "КонтрольДостоверностиОткрЗатВакуумного", "КонтрольДостоверностиЗакрЗатВакуумного", "КонтрольДостоверностиСостоянияСапуна", "КонтрольДостоверностиСостоянияУстройстваПлавПуска", "КонтрольДостоверностиСостоянияПитанияВакуумногоНасоса", "КонтрольДостоверностиСостоянияПитанияВентилятора", "КонтрольДостоверностиСостоянияПитанияРегТемпературы", "КонтрольДостоверностиСостоянияПитанияРегУровня", "КонтрольДостоверностиУровняВодыМинимум", "КонтрольДостоверностиУровняВодыМаксимум", "КонтрольДостоверностиСостоянияПитанияНасОхлаждения", "ЧтениеФактПараметров_с_Датчиков", "РЕГУЛЯТОР_ТРАФИКА", "ЧтениеКольцевогоБуфера", "ОбработкаКомандИзмененияНП_от_ГУИ", "ОбработкаКомандУправления_от_ГУИ", "КонтрольИзменения_ФП_P_ВбакеКомпрессора", "КонтрольИзменения_ФП_P_Впатрубке", "КонтрольИзменения_ФП_T_Врубашке", "КонтрольИзменения_ФП_T_Вбаке", "КонтрольИзменения_ФП_P_ВтрубеСидер", "КонтрольВеличиныОткачкиВауумнойТрубыСидеростата", "КонтрольГотовностиВакуума_в_Вакуумной_Трубе", "КонтрольУровняВодыБакаОхлаждения", "КонтрольТемпературыВодыБакаОхлаждения", "КонтрольТемпературыРубашкиОхлаждения", "КонтрольДавленияВбакеКомпрессора", "ВКЛ_ПИТ_ВЕНТИЛЯТОР", "ВЫК_ПИТ_ВЕНТИЛЯТОР", "КонтрольСостоянияПитанияВентилятора", "КонтрольСпонтанногоВыключенияВентилятора", "КонтрольСпонтанногоВключенияВентилятора", "КонтрольСостоянияЗатвораВакуумного", "ОТКР_ЗАТВОР_ВАК", "ЗАКР_ЗАТВОР_ВАК", "КонтрольСпонтанногоЗакрытияЗатвораВакуумного", "КонтрольСпонтанногоОткрытияЗатвораВакуумного", "ОТКР_САПУН", "ЗАКР_САПУН", "КонтрольСостоянияПитанияСапуна", "КонтрольСпонтанногоЗакрытияСапуна", "КонтрольСпонтанногоОткрытияСапуна", "ВКЛ_ПИТ_ВАК_НАСОСА", "ВЫК_ПИТ_ВАК_НАСОСА", "КонтрольСостоянияПитанияВакуумногоНасоса", "КонтрольСпонтанногоВыключенияВакНасоса", "КонтрольСпонтанногоВключенияВакНасоса", "ВКЛ_ПИТ_РЕГ_Т", "ВЫК_ПИТ_РЕГ_Т", "КонтрольСостоянияПитанияРЕГ_Т", "КонтрольСпонтанногоВыключенияРЕГ_Т", "КонтрольСпонтанногоВключенияРЕГ_Т", "ВКЛ_ПИТ_РЕГ_УР", "ВЫК_ПИТ_РЕГ_УР", "КонтрольСостоянияПитанияРЕГ_УР", "КонтрольСпонтанногоВыключенияРЕГ_УР", "КонтрольСпонтанногоВключенияРЕГ_УР", "ВКЛ_ПИТ_НАС_ОХЛ", "ВЫК_ПИТ_НАС_ОХЛ", "КонтрольСостоянияПитанияНАС_ОХЛ", "КонтрольСпонтанногоВыключенияНасосаОхлаждения", "КонтрольСпонтанногоВключенияНасосаОхлаждения", "ВКЛ_УСТР_ПЛАВ_ПУСКА", "ВЫК_УСТР_ПЛАВ_ПУСКА", "КонтрольСостоянияПитанияПЛАВ_ПУСКА", "КонтрольСпонтанногоВыключенияПлавнПуска", "КонтрольСпонтанногоВключенияПлавнПуска", "ВКЛ_ВАКУУМИРОВАНИЕ_ТРУБЫ", "ВЫК_ВАКУУМИРОВАНИЕ_ТРУБЫ", "ВКЛ_ВАКУУМНУЮ_ПОДСИСТЕМУ", "ВЫК_ВАКУУМНУЮ_ПОДСИСТЕМУ"]
  out "Init  VOC INPUT":u8[](array[numeric])
  out "Alg Input":i32[](array[numeric])=[2, 2, 2, 2, 2, 2, 2, 2, 2, 2, 2]
  out "Init ALG input":u8[](array[numeric])
  in  "stop":bool
  # "К_ОТКР_ЗАТВОР_ВАК"
  # "К_ЗАКР_ЗАТВОР_ВАК"
  # "У_ПИТ_ВЕНТИЛЯТОРА"
  # "К_САПУН"
  # "У_ПИТ_РЕГ_Т"
  # "К_УСТР_ПЛАВ_ПУСКА"
  # "У_ПИТ_НАС_ОХЛ"
  # "К_ПИТ_ВАК_НАСОСА"
  # "У_ПИТ_ВАК_НАСОСА"
  # "К_ВЕНТИЛЯТОР"
  # "У_ЗАТВОР_ВАК"
  # "К_ПИТ_РЕГ_Т"
  # "У_САПУН"
  # "К_ПИТ_РЕГ_УР"
  # "У_УСТР_ПЛАВ_ПУСКА"
  # "К_УР_ВОДЫ_MIN"
  # "У_ПИТ_РЕГ_УР"
  # "К_УР_ВОДЫ_MAX"
  # "К_ПИТ_НАСОС_ОХЛ"
  # "К_ЛОГ_ВХОД_P_ВбакеКомпрессора"
  # "К_ЛОГ_ВХОД_P_Впатрубке"
  # "К_ЛОГ_ВХОД_T_Врубашке"
  # "К_ЛОГ_ВХОД_T_Вбаке"
  # "К_ЛОГ_ВХОД_P_ВтрубеСидер"
  # "STEP MODE"
  # "CONTINUOUS MODE"
  # "ALG MSG Generation"
  # "VOC MSG Generation"
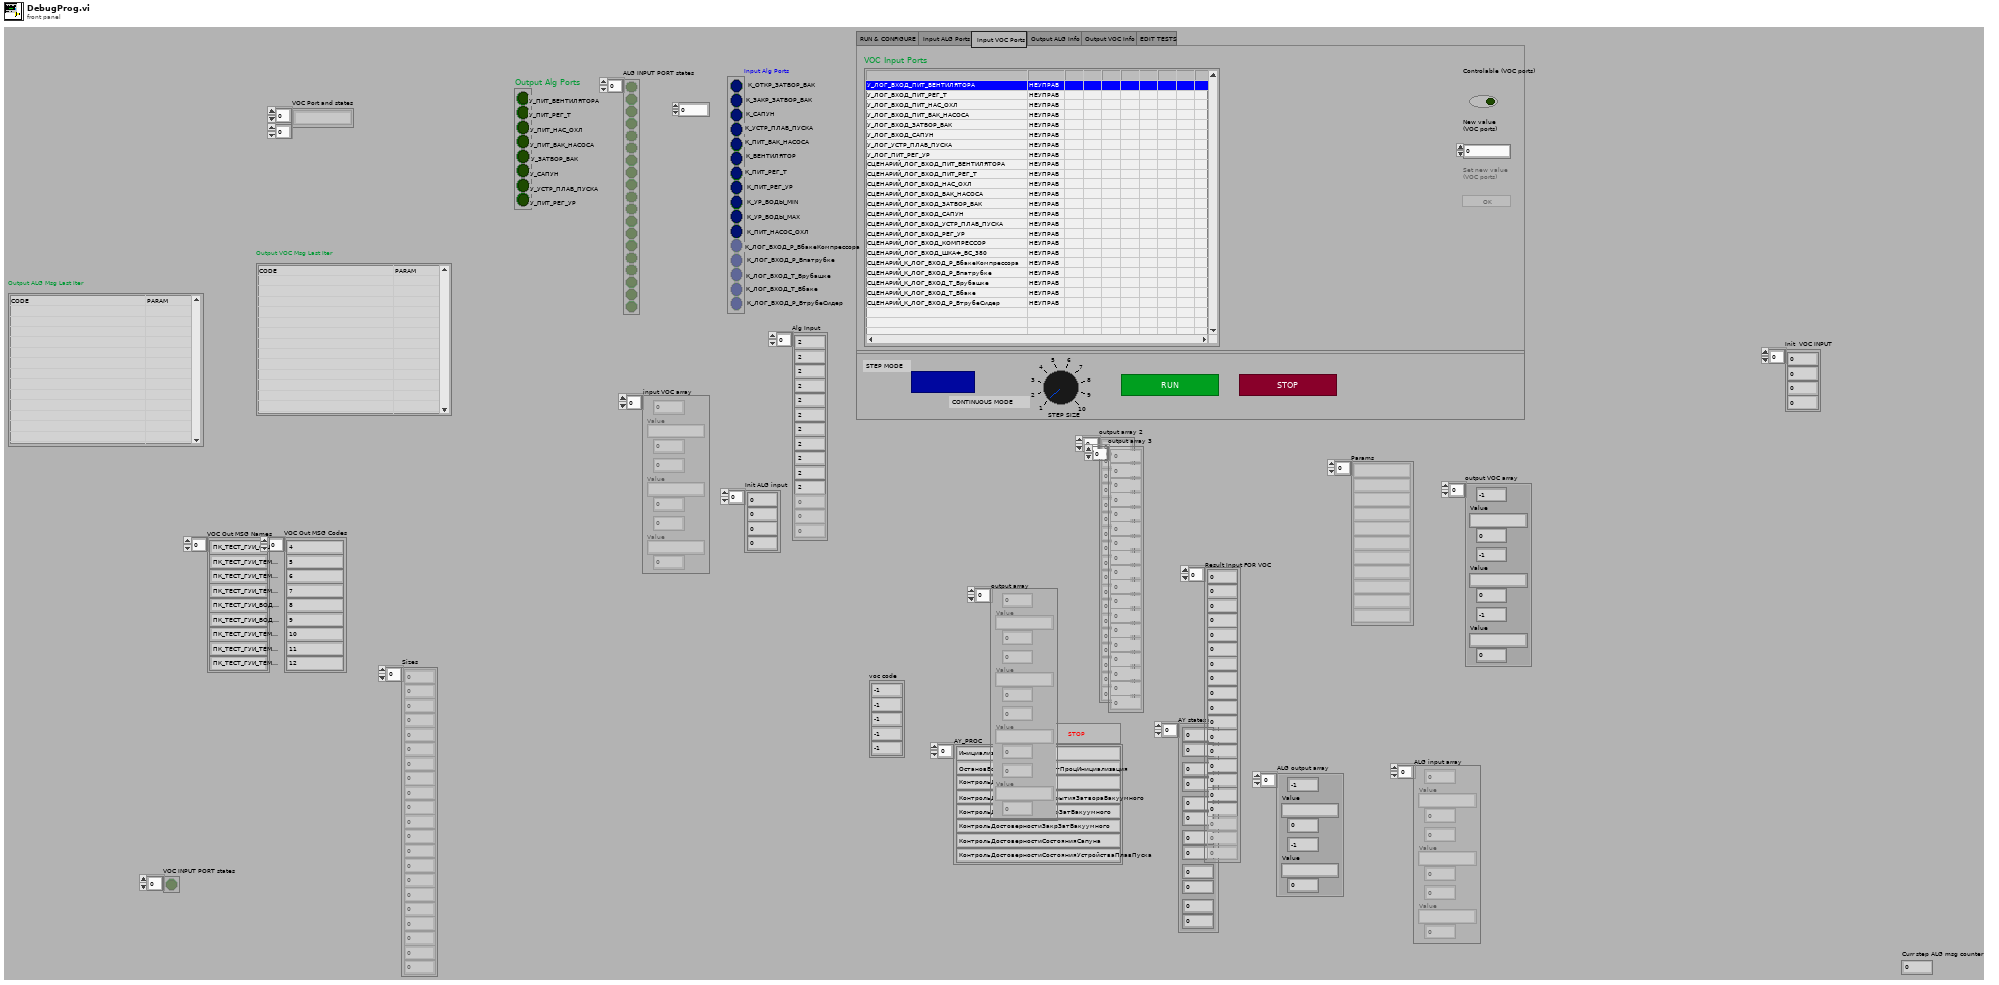
[diagram p1: front panel]
types:
  T1 = enum32{"RUN & CONFIGURE", "Input ALG Ports", "Input VOC Ports ", "Output ALG Info", "Output VOC Info", "EDIT TESTS"}
  T2 = enum16{"open", "open or create", "create or replace", "create", "open (read only)"}
  T3 = cluster{"trimmed string":string, "trimmed string":string}[]
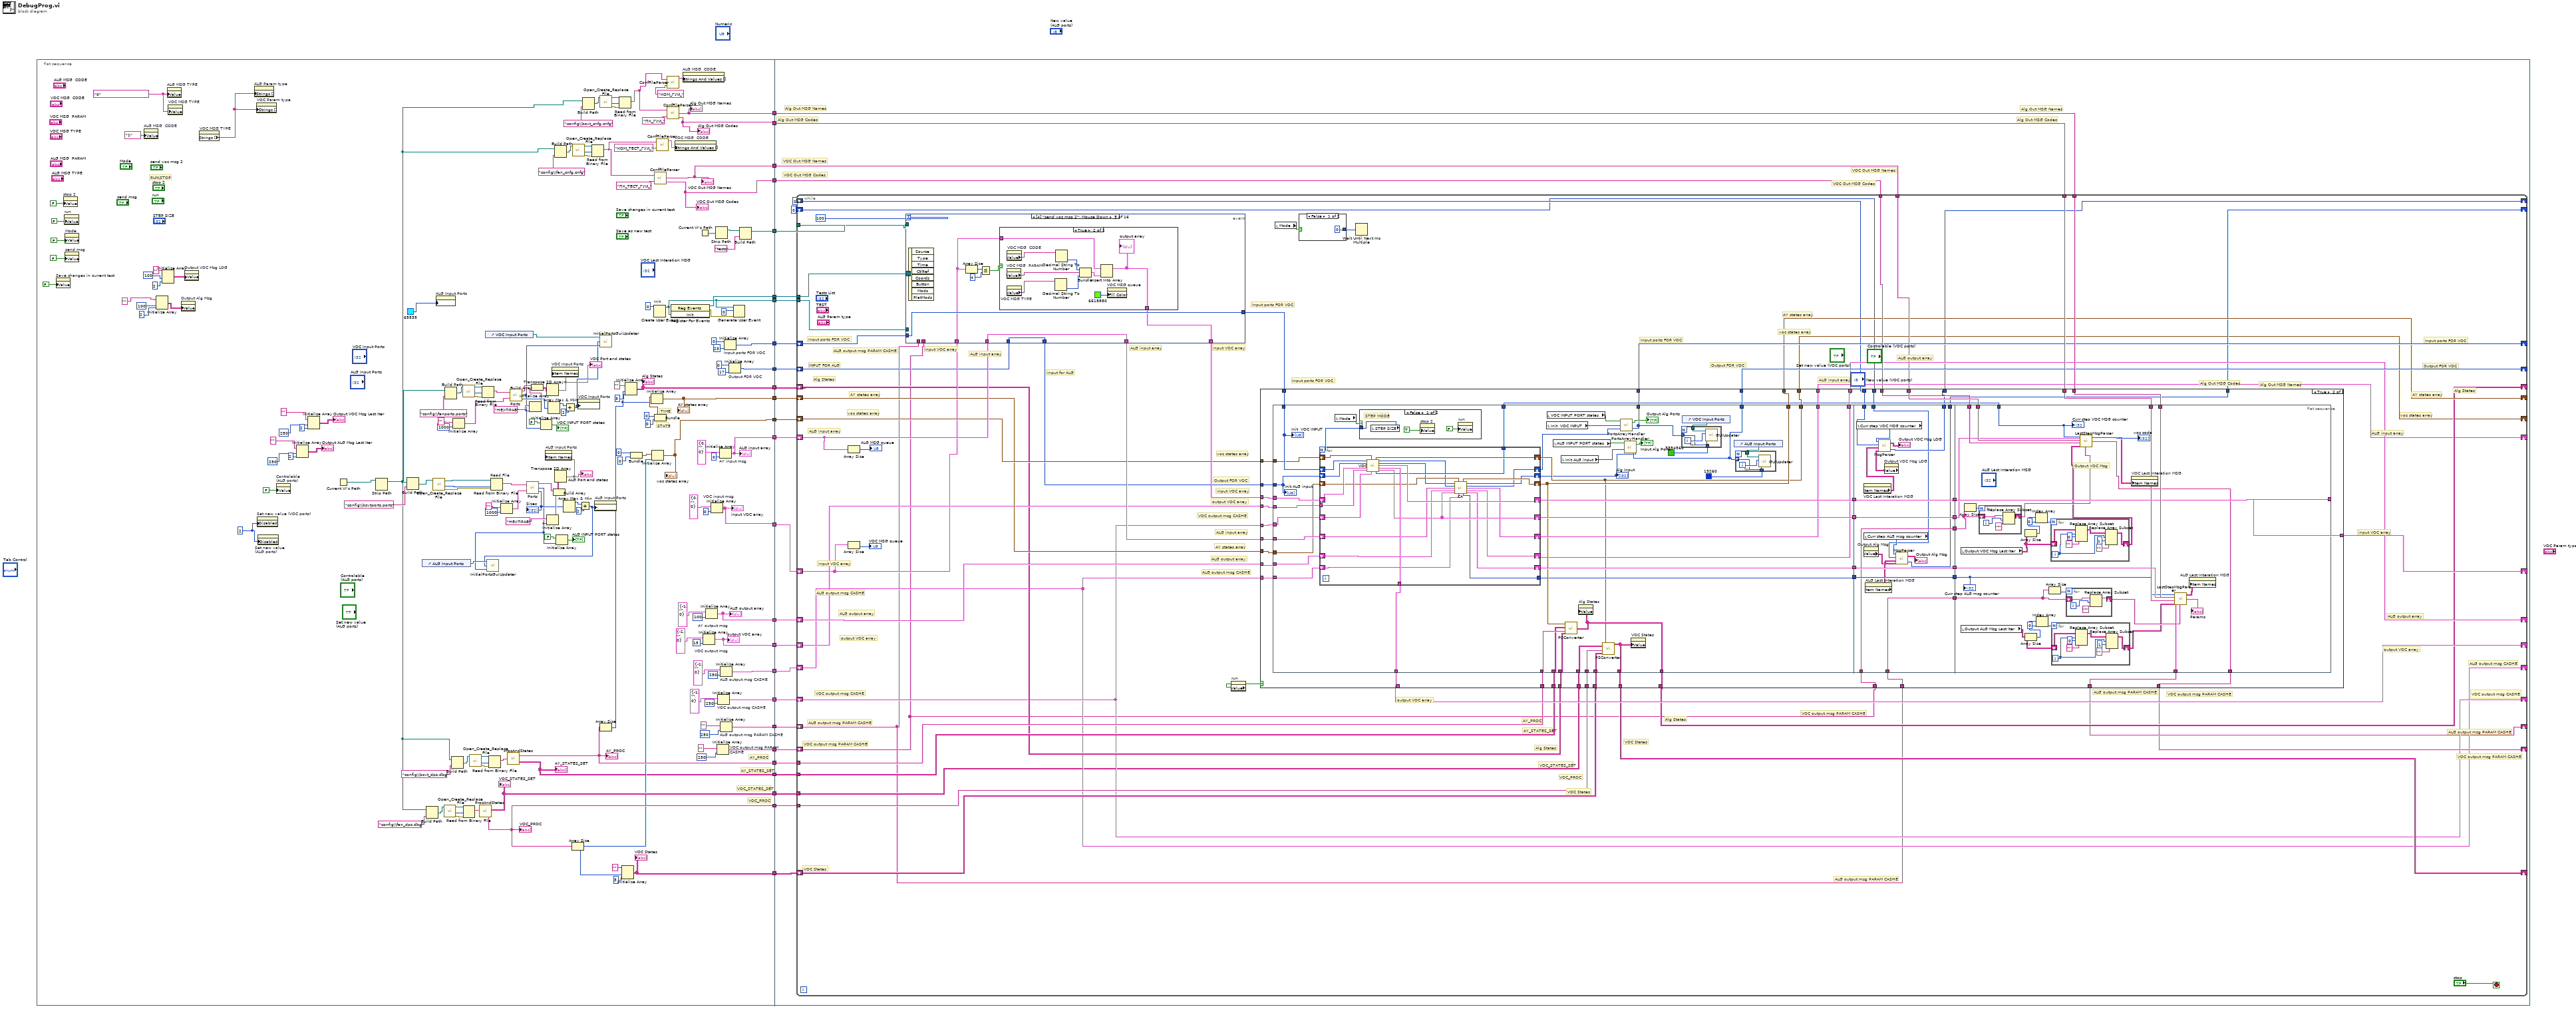
[diagram p0: block diagram]
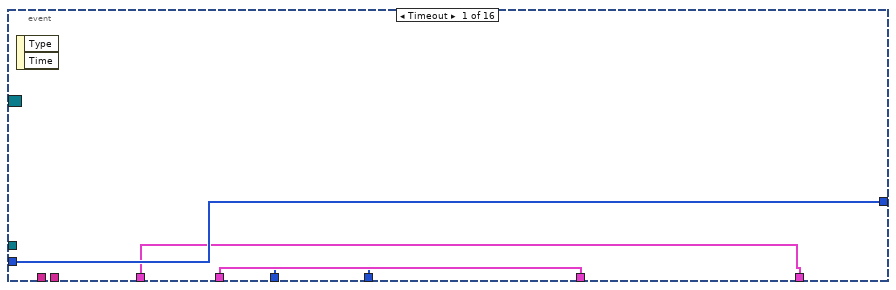
[diagram p2: hidden frame]
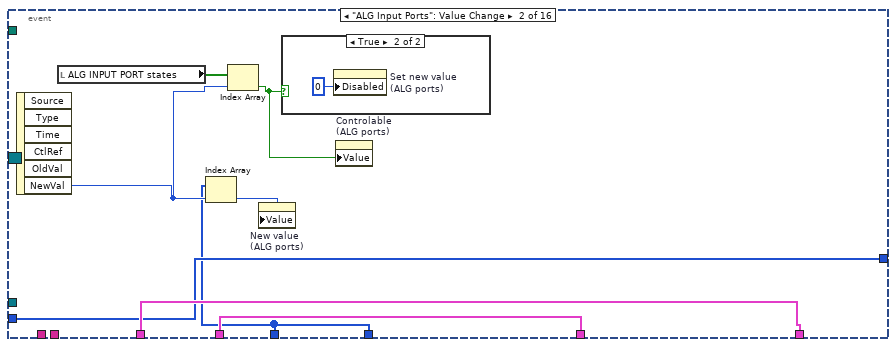
[diagram p3: hidden frame]
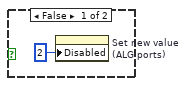
[diagram p4: hidden frame]
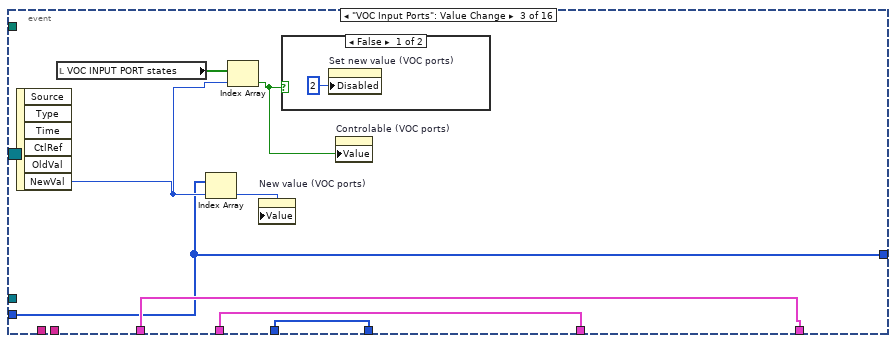
[diagram p5: hidden frame]
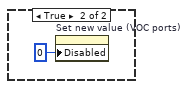
[diagram p6: hidden frame]
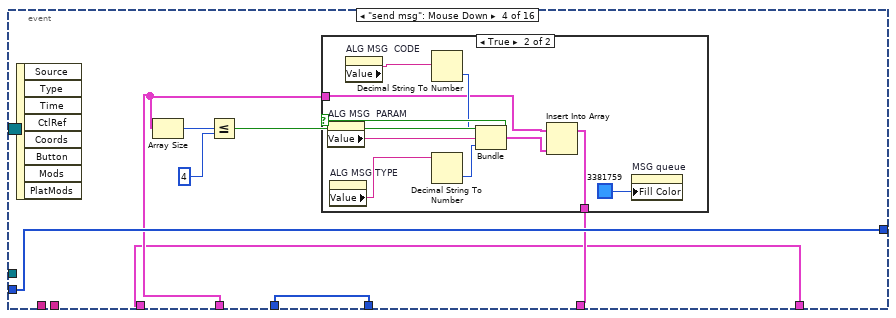
[diagram p7: hidden frame]
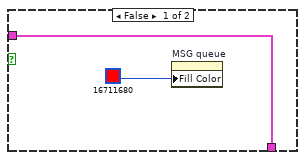
[diagram p8: hidden frame]
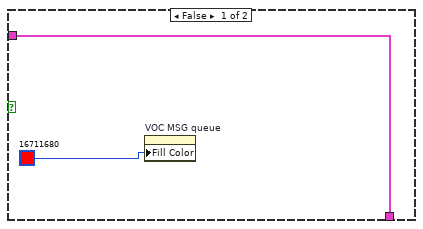
[diagram p9: hidden frame]
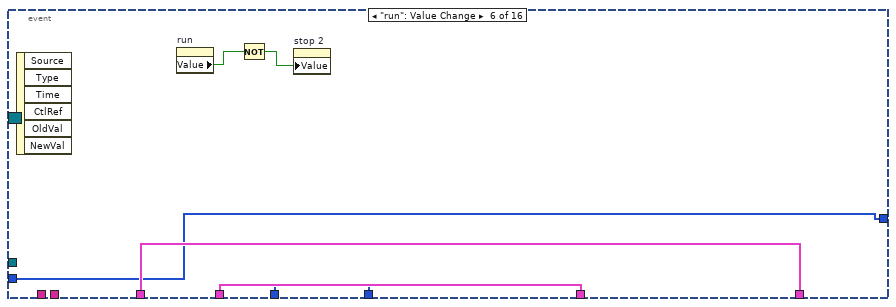
[diagram p10: hidden frame]
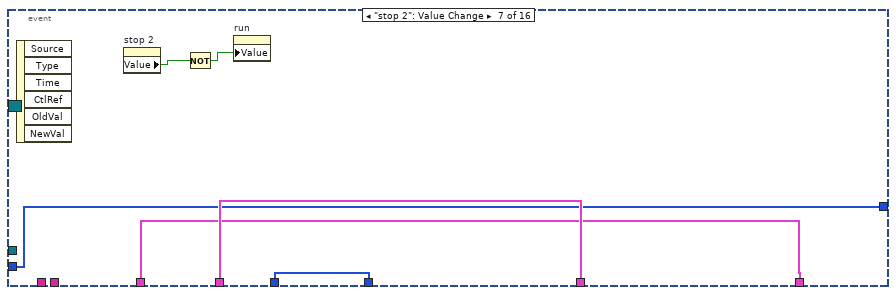
[diagram p11: hidden frame]
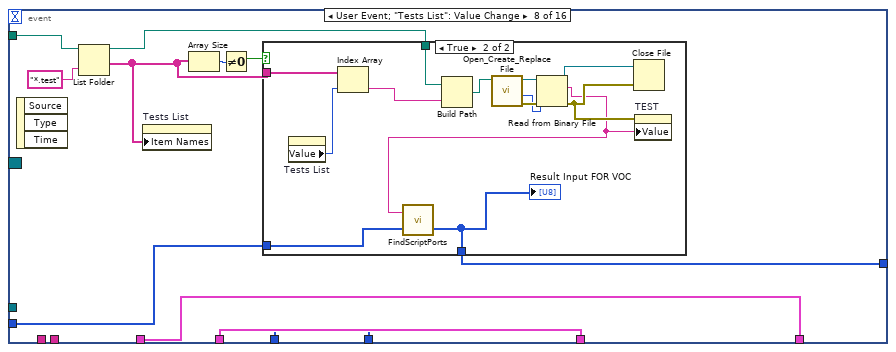
[diagram p12: hidden frame]
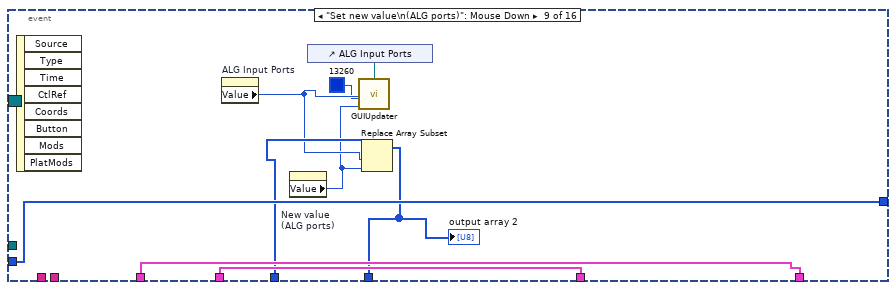
[diagram p14: hidden frame]
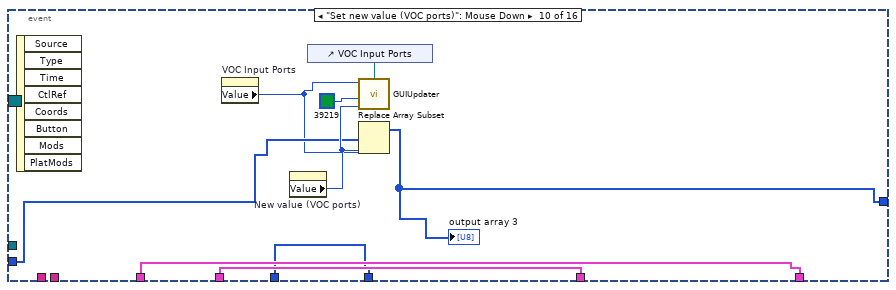
[diagram p15: hidden frame]
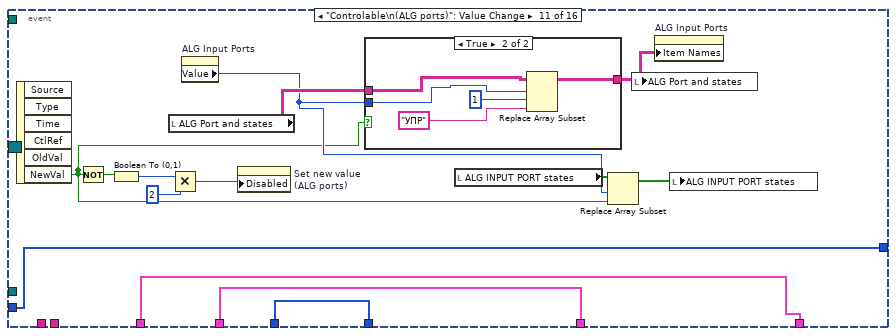
[diagram p16: hidden frame]
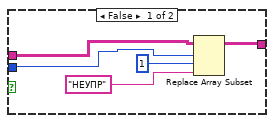
[diagram p17: hidden frame]
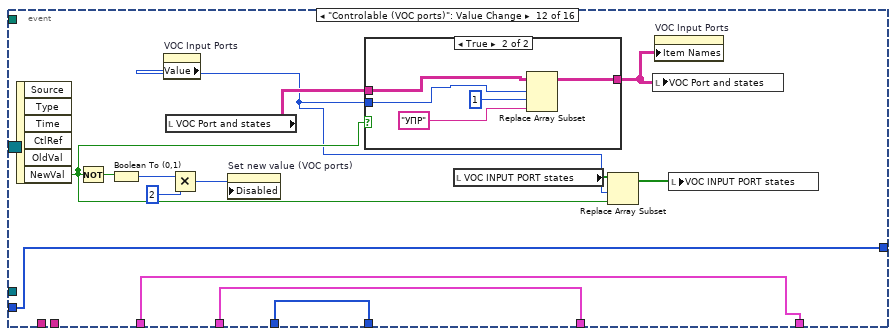
[diagram p18: hidden frame]
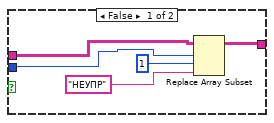
[diagram p19: hidden frame]
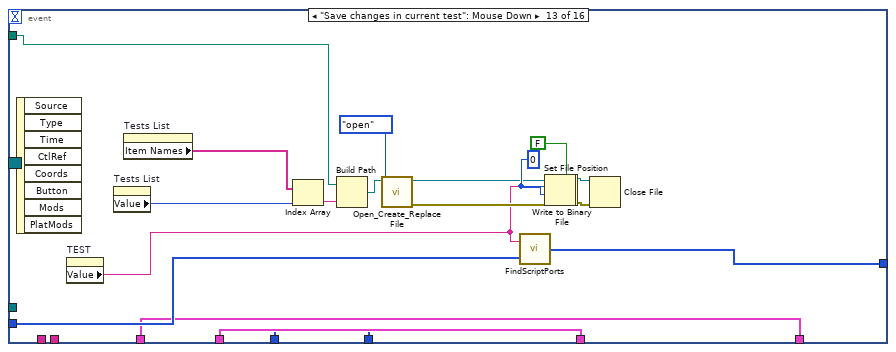
[diagram p20: hidden frame]
diagram:
  n1 = flat-sequence {
    tunnel: [w136] -> w25
    tunnel: [w128] -> w24
    tunnel: [w132] -> w23
    tunnel: [w129] -> w22
    tunnel: [w127] -> w21
    tunnel: [w126] -> w20
    tunnel: [w125] -> w19
    tunnel: [w123] -> w18
    tunnel: [w122] -> w17
    tunnel: [w121] -> w16
    tunnel: [w120] -> w15
    tunnel: [w117] -> w14
    tunnel: [w114] -> w13
    tunnel: [w113] -> w12
    tunnel: [w112] -> w11
    tunnel: [w111] -> w10
    tunnel: [w110] -> w9
    tunnel: [w96] -> w8
    tunnel: [w88] -> w7
    tunnel: [w90] -> w6
    tunnel: [w95] -> w5
    tunnel: [w94] -> w4
    tunnel: [w93] -> w3
    tunnel: [w85] -> w2
    tunnel: [w82] -> w1
    tunnel: w25 -> [w218]
    tunnel: w24 -> [w217]
    tunnel: w23 -> [w216]
    tunnel: w22 -> [w215]
    tunnel: w21 -> [w214]
    tunnel: w20 -> [w213]
    tunnel: w19 -> [w212]
    tunnel: w18 -> [w211]
    tunnel: w17 -> [w210]
    tunnel: w16 -> [w209]
    tunnel: w15 -> [w208]
    tunnel: w14 -> [w207]
    tunnel: w13 -> [w206]
    tunnel: w12 -> [w203]
    tunnel: w11 -> [w202]
    tunnel: w10 -> [w205]
    tunnel: w9 -> [w204]
    tunnel: w8 -> [w200]
    tunnel: w7 -> [w199]
    tunnel: w6 -> [w198]
    tunnel: w5 -> [w197]
    tunnel: w4 -> [w196]
    tunnel: w3 -> [w195]
    tunnel: w2 -> [w193]
    tunnel: w1 -> [w192]
    frame #0 {
      w27 = u8 2 ("Disabled")
      w135 = 0  # Init
      w181 = "0" ("TYPE")
      # "VOC_STATES_SET"
      # "VOC_PROC"
      # "AY_STATES_SET"
      # "AY_PROC"
      # "STATE"
      # "TIME"
      # "RUN\\STOP"
      n2 = property on="Save changes in current test" class="Bool (strict)"("Value"=FALSE ("Save changes in current test")) -> ()  [unwired: 2 in, 2 out]
      n3 = property on="stop 2" class="Bool (strict)"("Value"=FALSE ("send msg 3")) -> ()  [unwired: 2 in, 2 out]
      n4 = property on="run" class="Bool (strict)"("Value"=FALSE ("send msg 2")) -> ()  [unwired: 2 in, 2 out]
      n5 = property on="Mode" class="Bool (strict)"("Value"=FALSE ("Mode")) -> ()  [unwired: 2 in, 2 out]
      n6 = property on="send msg" class="Bool (strict)"("Value"=FALSE ("send msg")) -> ()  [unwired: 2 in, 2 out]
      n7 = property on="ALG MSG  CODE" class="CmbBox"("Value"="1" ("CODE")) -> ()  [unwired: 2 in, 2 out]
      n8 = Initialize Array("" ("element"), 100 ("dimension size"), 2 ("dimension size")) -> (w101:string[][])
      n9 = Initialize Array("" ("element"), 100 ("dimension size"), 2 ("dimension size")) -> (w102:string[][])
      n10 = property on="ALG MSG TYPE" class="CmbBox"("Value"=w181) -> ()  [unwired: 2 in, 2 out]
      n11 = property on="VOC MSG TYPE" class="CmbBox"("Value"=w181) -> ()  [unwired: 2 in, 2 out]
      n12 = property on="Output Alg Msg" class="Tbl (strict)"("Value"=w101) -> ()  [unwired: 2 in, 2 out]
      n13 = property on="Output VOC Msg LOG" class="Tbl (strict)"("Value"=w102) -> ()  [unwired: 2 in, 2 out]
      n14 = property on="VOC MSG TYPE" class="CmbBox"() -> ("Strings []"=w178:string[])  [unwired: 2 in, 2 out]
      n15 = property on="ALG Param type" class="CmbBox"("Strings []"=w178) -> ()  [unwired: 2 in, 2 out]
      n16 = property on="VOC Param type" class="CmbBox"("Strings []"=w178) -> ()  [unwired: 2 in, 2 out]
      n17 = property on="Set new value (VOC ports)" class="Bool (strict)"("Disabled"=w27) -> ()  [unwired: 2 in, 2 out]
      n18 = property on="Set new value\n(ALG ports)" class="Bool (strict)"("Disabled"=w27) -> ()  [unwired: 2 in, 2 out]
      n19 = property on="Controlable\n(ALG ports)" class="Bool (strict)"("Value"=FALSE ("Controlable")) -> ()  [unwired: 2 in, 2 out]
      n20 = Initialize Array("" ("Value"), 250 ("dimension size"), 2 ("dimension size")) -> (→"Output ALG Msg Last Iter":string[][])
      n21 = Initialize Array("" ("Value"), 250 ("dimension size"), 2 ("dimension size")) -> (→"Output VOC Msg Last Iter":string[][])
      n22 = Current VI's Path() -> (path=w109:path)
      n23 = Strip Path(path=w109) -> (stripped path=w46:path)  [unwired: 1 out]
      n24 = Build Path(base path=w46, name or relative path="config\\bsvtports.ports") -> (appended path=w73:path)
      n25 = control-ref of="ALG Input Ports"() -> (w34:refnum<vi>)
      n26 = Build Path(base path=w46, name or relative path="config\\fan_dps.dbg") -> (appended path=w158:path)
      n27 = call <vilib>:"Open_Create_Replace File.vi"("file path"=w73) -> ("error out"=w72:errorcluster, "file size (bytes)"=w71:i32, "refnum"=w70:refnum<file>)  [unwired: 7 in, 1 out]
      n28 = property on="ALG Input Ports" class="MCListbox (strict)"("Selection Color"=u32 65535) -> ()  [unwired: 2 in, 2 out]
      n29 = call <vilib>:"Open_Create_Replace File.vi"("file path"=w158) -> ("error out"=w157:errorcluster, "file size (bytes)"=w156:i32, "refnum"=w155:refnum<file>)  [unwired: 7 in, 1 out]
      n30 = Build Path(base path=w46, name or relative path="config\\fanports.ports") -> (appended path=w53:path)
      n31 = Build Path(base path=w46, name or relative path="config\\bsvt_dps.dbg") -> (appended path=w150:path)
      n32 = Initialize Array("" ("name or relative path"), 1000 ("dimension size")) -> (w44:string[])
      n33 = call <vilib>:"Open_Create_Replace File.vi"("file path"=w53) -> ("error out"=w52:errorcluster, "file size (bytes)"=w51:i32, "refnum"=w50:refnum<file>)  [unwired: 7 in, 1 out]
      n34 = Read from Binary File(8:w157, 10:w156, 11:w155) -> (2:w124:string)  [unwired: 3 in, 3 out]
      n35 = call <vilib>:"Open_Create_Replace File.vi"("file path"=w150) -> ("error out"=w149:errorcluster, "file size (bytes)"=w148:i32, "refnum"=w147:refnum<file>)  [unwired: 7 in, 1 out]
      n36 = call "ProcAndStates.vi"("spreadsheet string"=w124) -> ("PROCESSES"=w90:string[], "STATES"=w95:string[][])
      "VOC_PROC" <- w90
      "VOC_STATES_SET" <- w95
      n37 = Read from Binary File(8:w52, 10:w51, 11:w50) -> (2:w45:string)  [unwired: 3 in, 3 out]
      n38 = control-ref of="VOC Input Ports"() -> (w31:refnum<vi>)
      n39 = Read from Binary File(8:w149, 10:w148, 11:w147) -> (2:w160:string)  [unwired: 3 in, 3 out]
      n40 = Read from Binary File "Read File"(8:w72, 10:w71, 11:w70) -> (2:w66:string)  [unwired: 3 in, 3 out]
      n41 = Initialize Array("" ("name or relative path"), 1000 ("dimension size")) -> (w65:string[])
      n42 = call "ProcAndStates.vi"("spreadsheet string"=w160) -> ("PROCESSES"=w96:string[], "STATES"=w88:string[][])
      "AY_PROC" <- w96
      "AY_STATES_SET" <- w88
      n43 = call "Ports.vi"("Test"=w45, "Reserved array Input"=w44) -> ("Result Input"=w42:string[], "Ports counter"=w30:i32, "Sizes"=w37:i32[])
      n44 = call "Ports.vi"("Test"=w66, "Reserved array Input"=w65) -> ("Result Input"=w54:string[], "Ports counter"=w33:i32, "Sizes"=w57:i32[])
      "Sizes" <- w57
      n45 = Initialize Array("НЕУПРАВ" ("name or relative path"), w30) -> (w41:string[])
      n46 = Build Array(w42, w41) -> (w40:string[][])
      n47 = Initialize Array(FALSE, w30) -> (→"VOC INPUT PORT states":bool[])
      n48 = Initialize Array("НЕУПРАВ" ("name or relative path"), w33) -> (w62:string[])
      n49 = Transpose 2D Array(2D array=w40) -> (transposed array=w28:string[][])
      "VOC Port and states" <- w28
      n50 = Array Max & Min(array=w37) -> (max value=w39:i32)  [unwired: 3 out]
      n51 = property on="VOC Input Ports" class="MCListbox (strict)"("Item Names"=w28) -> ()  [unwired: 2 in, 2 out]
      n52 = Build Array(w54, w62) -> (w63:string[][])
      n53 = Build Path(base path=w46, name or relative path="config\\fan_cnfg.cnfg") -> (appended path=w174:path)
      n54 = Transpose 2D Array(2D array=w63) -> (transposed array=w61:string[][])
      "ALG Port and states" <- w61
      n55 = property on="ALG Input Ports" class="MCListbox (strict)"("Item Names"=w61) -> ()  [unwired: 2 in, 2 out]
      n56 = Initialize Array(FALSE, w33) -> (→"ALG INPUT PORT states":bool[])
      n57 = Array Max & Min(array=w57) -> (max value=w56:i32)  [unwired: 3 out]
      n58 = Add(x=w39, y=2) -> (x+y=w29:i32)
      n59 = Array Size(array=w90) -> (size(s)=w89:i32)
      n60 = call <vilib>:"Open_Create_Replace File.vi"("file path"=w174) -> ("error out"=w173:errorcluster, "file size (bytes)"=w172:i32, "refnum"=w171:refnum<file>)  [unwired: 7 in, 1 out]
      n61 = property on="VOC Input Ports" class="MCListbox (strict)"("Number of Columns"=w29) -> ()  [unwired: 2 in, 2 out]
      n62 = Add(x=w56, y=2) -> (x+y=w32:i32)
      n63 = call "InitialPortsGuiUpdater.vi"("Ports counter"=w33, "port max size"=w32, "MCListbox Refnum"=w34) -> ()
      n64 = Build Path(base path=w46, name or relative path="config\\bsvt_cnfg.cnfg") -> (appended path=w146:path)
      n65 = Read from Binary File(8:w173, 10:w172, 11:w171) -> (2:w176:string)  [unwired: 3 in, 3 out]
      n66 = property on="ALG Input Ports" class="MCListbox (strict)"("Number of Columns"=w32) -> ()  [unwired: 2 in, 2 out]
      n67 = Array Size(array=w96) -> (size(s)=w104:i32)
      n68 = call <vilib>:"Open_Create_Replace File.vi"("file path"=w146) -> ("error out"=w145:errorcluster, "file size (bytes)"=w144:i32, "refnum"=w143:refnum<file>)  [unwired: 7 in, 1 out]
      n69 = call "InitialPortsGuiUpdater.vi"("Ports counter"=w30, "port max size"=w29, "MCListbox Refnum"=w31) -> ()
      n70 = Read from Binary File(8:w145, 10:w144, 11:w143) -> (2:w167:string)  [unwired: 3 in, 3 out]
      n71 = Initialize Array("" ("Value"), w89, 3 ("dimension size")) -> (w93:string[][])
      "VOC States" <- w93
      n72 = Initialize Array("" ("Value"), w104, 3 ("dimension size")) -> (w94:string[][])
      "Alg States" <- w94
      n73 = Bundle(u32 0, u8 0) -> (w166:cluster{u32, u8})  [unwired: 1 in]
      n74 = Initialize Array(w166, w89) -> (w122:cluster{u32, u8}[])
      "voc states array" <- w122
      n75 = Create User Event(user event datatype=w135) -> (user event=w128:refnum<user-event>)  [unwired: 1 in, 1 out]
      n76 = call "ConfFileParser.vi"("TEXT"=w176, "search string"="ПК_ТЕСТ_ГУИ_") -> ("Names"=w111:string[], "Codes"=w110:string[])  [unwired: 1 out]
      "VOC Out MSG Names" <- w111
      "VOC Out MSG Codes" <- w110
      n77 = Bundle(u32 0, u8 0) -> (w163:cluster{u32, u8})  [unwired: 1 in]
      n78 = Initialize Array(w163, w104) -> (w123:cluster{u32, u8}[])
      "AY states array" <- w123
      n79 = call "ConfFileParser.vi"("TEXT"=w176, "search string"="КОМ_ТЕСТ_ГУИ_") -> ("Cluster Array"=w169:T3)  [unwired: 2 out]
      n80 = call "ConfFileParser.vi"("TEXT"=w167, "search string"="КОМ_ГУИ_") -> ("Cluster Array"=w152:T3)  [unwired: 2 out]
      n81 = call "ConfFileParser.vi"("TEXT"=w167, "search string"="ПК_ГУИ_") -> ("Names"=w113:string[], "Codes"=w112:string[])  [unwired: 1 out]
      "Alg Out MSG Names" <- w113
      "Alg Out MSG Codes" <- w112
      n82 = register-events(w128) -> (reference out=w132:refnum<event-registration>, error out=w134:errorcluster)  [unwired: 2 in]
      n83 = property on="VOC MSG  CODE" class="CmbBox"("Strings And Values []"=w169) -> ()  [unwired: 2 in, 2 out]
      n84 = property on="ALG MSG  CODE" class="CmbBox"("Strings And Values []"=w152) -> ()  [unwired: 2 in, 2 out]
      n85 = Current VI's Path() -> (path=w138:path)
      n86 = Initialize Array "VOC output msg"(cluster{i32, "Value":string, i32} {-1, "Value"="", 0} ("element"), 15 ("dimension size")) -> (w120:cluster{i32, "Value":string, i32}[])
      "output VOC array" <- w120
      n87 = Initialize Array "AY output msg"(cluster{i32, "Value":string, i32} {-1, "Value"="", 0} ("element"), 100 ("dimension size")) -> (w121:cluster{i32, "Value":string, i32}[])
      "ALG output array" <- w121
      n88 = Initialize Array "VOC input msg"(cluster{i32, "Value":string, i32} {0, "Value"="", 0} ("element"), 0 ("dimension size")) -> (w126:cluster{i32, "Value":string, i32}[])
      "input VOC array" <- w126
      n89 = Strip Path(path=w138) -> (stripped path=w137:path)  [unwired: 1 out]
      n90 = Initialize Array "VOC output msg PARAM CASHE"("" ("Value"), 250 ("dimension size")) -> (w82:string[])
      n91 = Initialize Array "VOC output msg CASHE"(cluster{i32, "Value":string, i32} {-1, "Value"="", 0} ("element"), 250 ("dimension size")) -> (w117:cluster{i32, "Value":string, i32}[])
      n92 = Initialize Array "AY input msg"(cluster{i32, "Value":string, i32} {0, "Value"="", 0} ("element"), 0 ("dimension size")) -> (w127:cluster{i32, "Value":string, i32}[])
      "ALG input array" <- w127
      n93 = Initialize Array "ALG output msg PARAM CASHE"("" ("Value"), 250 ("dimension size")) -> (w85:string[])
      n94 = Initialize Array "ALG output msg CASHE"(cluster{i32, "Value":string, i32} {-1, "Value"="", 0} ("element"), 250 ("dimension size")) -> (w114:cluster{i32, "Value":string, i32}[])
      n95 = Initialize Array "Input ports FOR VOC"(u8 0 ("element"), 23 ("dimension size")) -> (w129:u8[])
      n96 = Initialize Array "Output FOR VOC"(u8 0 ("element"), 17 ("dimension size")) -> (w125:u8[])
      n97 = Generate User Event(user event=w128, event data cluster=0, error in=w134) -> ()  [unwired: 2 out]
      n98 = Build Path(base path=w137, name or relative path="tests") -> (appended path=w136:path)
    }
    frame #1 {
      # "VOC Out MSG Names"
      # "Alg Out MSG Codes"
      # "Alg Out MSG Names"
      # "VOC Out MSG Codes"
      # "VOC Out MSG Codes"
      # "VOC Out MSG Names"
      # "Alg Out MSG Codes"
      # "Alg Out MSG Names"
      n99 = while {
        tunnel: w218 -> [w261]
        tunnel: w217 -> [w264]
        tunnel: w216 -> [w265]
        shift-right: [w248] -> _
        shift-left: w215 -> [w263]
        shift-right: [w227] -> _
        shift-left: w214 -> [w260]
        shift-right: [w242] -> _
        shift-left: w213 -> [w245]
        shift-right: [w247] -> _
        shift-left: w212 -> [w220]
        shift-right: [w246] -> _
        shift-left: w211 -> [w255]
        shift-right: [w226] -> _
        shift-left: w210 -> [w256]
        shift-right: [w244] -> _
        shift-left: w209 -> [w254]
        shift-right: [w243] -> _
        shift-left: w208 -> [w253]
        shift-right: [w229] -> _
        shift-left: w207 -> [w229]
        shift-right: [w228] -> _
        shift-left: w206 -> [w228]
        tunnel: w205 -> [w252]
        tunnel: w204 -> [w251]
        tunnel: w203 -> [w249]
        tunnel: w202 -> [w250]
        shift-right: [w239] -> _
        shift-left: 0 -> [w240]
        tunnel: w198 -> [w236]
        tunnel: w200 -> [w238]
        tunnel: w199 -> [w237]
        tunnel: w197 -> [w225]
        shift-right: [w234] -> _
        shift-left: w196 -> [w235]
        shift-right: [w232] -> _
        shift-left: w195 -> [w233]
        shift-right: [w230] -> _
        shift-left: 0 -> [w231]
        shift-right: [w224] -> _
        shift-left: w193 -> [w223]
        shift-right: [w221] -> _
        shift-left: w192 -> [w222]
        stop <- "stop" stop-if-true
        # "Input for ALG"
        # "VOC output msg PARAM CASHE"
        # "VOC output msg PARAM CASHE"
        # "VOC output msg PARAM CASHE"
        # "VOC output msg PARAM CASHE"
        # "ALG output msg PARAM CASHE"
        # "ALG output msg PARAM CASHE"
        # "ALG output msg PARAM CASHE"
        # "ALG output msg PARAM CASHE"
        # "ALG output msg PARAM CASHE"
        # "voc states array"
        # "VOC States"
        # "Alg States"
        # "VOC States"
        # "VOC States"
        # "Alg States"
        # "Alg States"
        # "Alg States"
        # "VOC_STATES_SET"
        # "VOC_PROC"
        # "AY_STATES_SET"
        # "AY_PROC"
        # "output VOC array"
        # "AY states array"
        # "ALG output array"
        # "ALG input array"
        # "ALG output msg CASHE"
        # "VOC output msg CASHE"
        # "output VOC array"
        # "ALG output array"
        # "input VOC array"
        # "ALG input array"
        # "voc states array"
        # "AY states array"
        # "Output FOR VOC"
        # "Input ports FOR VOC"
        # "Output FOR VOC"
        # "Input ports FOR VOC"
        # "Alg Out MSG Codes"
        # "Alg Out MSG Names"
        # "ALG output msg CASHE"
        # "ALG output msg CASHE"
        # "VOC output msg CASHE"
        # "VOC output msg CASHE"
        # "ALG output array"
        # "output VOC array"
        # "output VOC array"
        # "ALG output array"
        # "AY states array"
        # "voc states array"
        # "voc states array"
        # "AY states array"
        # "ALG input array"
        # "Output FOR VOC"
        # "INPUT FOR ALG"
        # "input VOC array"
        # "Input ports FOR VOC"
        # "input VOC array"
        # "ALG input array"
        # "input VOC array"
        # "input VOC array"
        # "Input ports FOR VOC"
        # "Input ports FOR VOC"
        # "ALG input array"
        # "ALG input array"
        n100 = Array Size(array=w260) -> (size(s)=→"ALG MSG queue":i32)
        n101 = Array Size(array=w245) -> (size(s)=→"VOC MSG queue":i32)
        n102 = event shown="[4] \"send voc msg 2\": Mouse Down" {
          selector: w265 -> [_ _ _ _ _ _ _ _ _ _ _ _ _ _ _ _]
          dyn-events: _ -> [_ _ _ _ _ _ _ _ _ _ _ _ _ _ _ _]
          timeout: 100 -> [_ _ _ _ _ _ _ _ _ _ _ _ _ _ _ _]
          tunnel: w263 -> [w274 w278 w285 w302 w320 w334 w340 w353 w376 w383 w399 w423 w451 w465 w477 w502]
          tunnel: w264 -> [_ _ _ _ _ _ _ _ _ _ _ _ _ _ _ _]
          tunnel: [w274 w278 w285 w302 w320 w334 w340 w352 w376 w381 w399 w423 w450 w465 w477 w501] -> w259
          tunnel: w261 -> [_ _ _ _ _ _ _ w349 _ _ _ _ w449 _ _ w500]
          tunnel: w260 -> [w273 w282 w292 w298 w321 w336 w342 w347 w378 w387 w401 w425 w447 w467 w479 w499]
          tunnel: [w273 w282 w292 w297 w321 w336 w342 w347 w378 w387 w401 w425 w447 w467 w479 w499] -> w257
          tunnel: w245 -> [w272 w281 w291 w296 w316 w335 w341 w346 w377 w386 w400 w424 w446 w466 w478 w498]
          tunnel: [w272 w281 w291 w296 w315 w335 w341 w346 w377 w386 w400 w424 w446 w466 w478 w498] -> w258
          tunnel: w223 -> [_ _ _ _ _ _ _ _ _ _ _ _ _ w460 _ _]
          tunnel: w222 -> [_ _ _ _ _ _ _ _ _ _ _ _ _ _ w486 _]
          tunnel: w220 -> [w271 w277 w288 w295 w314 w333 w339 w345 w375 w382 w398 w422 w439 w456 w476 w496]
          tunnel: [w271 w277 w288 w295 w314 w333 w339 w345 w374 w382 w398 w422 w439 w456 w476 w496] -> w219
          event Timeout {
            n103 = event-data() -> ()  [unwired: 1 in, 2 out]
          }
          event "ALG Input Ports": Value Change {
            n104 = event-data() -> ("NewVal"=w279:i32)  [unwired: 1 in, 5 out]
            n105 = local read "ALG INPUT PORT states"() -> (w280:bool[])
            n106 = Index Array(array=w277, index=w279) -> (element=w276:i32)
            n107 = Index Array(array=w280, index=w279) -> (element=w275:bool)
            n108 = property on="New value\n(ALG ports)" class="DigNum (strict)"("Value"=w276) -> ()  [unwired: 2 in, 2 out]
            n109 = case shown="True" w275 {
              frame False {
                n110 = property on="Set new value\n(ALG ports)" class="Bool (strict)"("Disabled"=u8 2) -> ()  [unwired: 2 in, 2 out]
              }
              frame True {
                n111 = property on="Set new value\n(ALG ports)" class="Bool (strict)"("Disabled"=u8 0) -> ()  [unwired: 2 in, 2 out]
              }
            }
            n112 = property on="Controlable\n(ALG ports)" class="Bool (strict)"("Value"=w275) -> ()  [unwired: 2 in, 2 out]
          }
          event "VOC Input Ports": Value Change {
            n113 = event-data() -> ("NewVal"=w289:i32)  [unwired: 1 in, 5 out]
            n114 = local read "VOC INPUT PORT states"() -> (w290:bool[])
            n115 = Index Array(array=w285, index=w289) -> (element=w287:i32)
            n116 = Index Array(array=w290, index=w289) -> (element=w286:bool)
            n117 = property on="New value (VOC ports)" class="DigNum (strict)"("Value"=w287) -> ()  [unwired: 2 in, 2 out]
            n118 = case shown="False" w286 {
              frame False {
                n119 = property on="Set new value (VOC ports)" class="Bool (strict)"("Disabled"=u8 2) -> ()  [unwired: 2 in, 2 out]
              }
              frame True {
                n120 = property on="Set new value (VOC ports)" class="Bool (strict)"("Disabled"=u8 0) -> ()  [unwired: 2 in, 2 out]
              }
            }
            n121 = property on="Controlable (VOC ports)" class="Bool (strict)"("Value"=w286) -> ()  [unwired: 2 in, 2 out]
          }
          event "send msg": Mouse Down {
            n122 = event-data() -> ()  [unwired: 1 in, 8 out]
            n123 = Array Size(array=w298) -> (size(s)=w301:i32)
            n124 = Less Or Equal?(x=w301, y=4) -> (x <= y?=w299:bool)
            n125 = case shown="True" w299 {
              tunnel: w298 -> [w303 w307]
              tunnel: [w303 w305] -> w297
              frame False {
                n126 = property on="MSG queue" class="Slide (strict)"("Fill Color"=u32 16711680) -> ()  [unwired: 2 in, 2 out]
              }
              frame True {
                n127 = property on="ALG MSG  PARAM" class="Str"() -> ("Value"=w312:string)  [unwired: 2 in, 2 out]
                n128 = property on="ALG MSG TYPE" class="CmbBox"() -> ("Value"=w310:string)  [unwired: 2 in, 2 out]
                n129 = property on="ALG MSG  CODE" class="CmbBox"() -> ("Value"=w309:string)  [unwired: 2 in, 2 out]
                n130 = Decimal String To Number(string=w309) -> (number=w311:i32)  [unwired: 2 in, 1 out]
                n131 = Decimal String To Number(string=w310) -> (number=w313:i32)  [unwired: 2 in, 1 out]
                n132 = Bundle(w311, "Value"=w312, w313) -> (w306:cluster{i32, "Value":string, i32})  [unwired: 1 in]
                n133 = Insert Into Array(array=w307, new element=w306) -> (w305:cluster{i32, "Value":string, i32}[])  [unwired: 1 in]
                n134 = property on="MSG queue" class="Slide (strict)"("Fill Color"=u32 3381759) -> ()  [unwired: 2 in, 2 out]
              }
            }
          }
          event "send voc msg 2": Mouse Down {
            n135 = event-data() -> ()  [unwired: 1 in, 8 out]
            n136 = Array Size(array=w316) -> (size(s)=w317:i32)
            n137 = Less Or Equal?(x=w317, y=4) -> (x <= y?=w319:bool)
            n138 = case shown="True" w319 {
              tunnel: w316 -> [w322 w330]
              tunnel: [w322 w324] -> w315
              frame False {
                n139 = property on="VOC MSG queue" class="Slide (strict)"("Fill Color"=u32 16711680) -> ()  [unwired: 2 in, 2 out]
              }
              frame True {
                n140 = property on="VOC MSG  PARAM" class="Str"() -> ("Value"=w328:string)  [unwired: 2 in, 2 out]
                n141 = property on="VOC MSG  CODE" class="CmbBox"() -> ("Value"=w329:string)  [unwired: 2 in, 2 out]
                n142 = property on="VOC MSG TYPE" class="CmbBox"() -> ("Value"=w327:string)  [unwired: 2 in, 2 out]
                n143 = Decimal String To Number(string=w327) -> (number=w332:i32)  [unwired: 2 in, 1 out]
                n144 = Decimal String To Number(string=w329) -> (number=w331:i32)  [unwired: 2 in, 1 out]
                n145 = Bundle(w331, "Value"=w328, w332) -> (w325:cluster{i32, "Value":string, i32})  [unwired: 1 in]
                n146 = Insert Into Array(array=w330, new element=w325) -> (w324:cluster{i32, "Value":string, i32}[])  [unwired: 1 in]
                "output array" <- w324
                n147 = property on="VOC MSG queue" class="Slide (strict)"("Fill Color"=u32 6618880) -> ()  [unwired: 2 in, 2 out]
              }
            }
          }
          event "run": Value Change {
            n148 = event-data() -> ()  [unwired: 1 in, 6 out]
            n149 = property on="run" class="Bool (strict)"() -> ("Value"=w338:bool)  [unwired: 2 in, 2 out]
            n150 = Not(x=w338) -> (.not. x?=w337:bool)
            n151 = property on="stop 2" class="Bool (strict)"("Value"=w337) -> ()  [unwired: 2 in, 2 out]
          }
          event "stop 2": Value Change {
            n152 = event-data() -> ()  [unwired: 1 in, 6 out]
            n153 = property on="stop 2" class="Bool (strict)"() -> ("Value"=w344:bool)  [unwired: 2 in, 2 out]
            n154 = Not(x=w344) -> (.not. x?=w343:bool)
            n155 = property on="run" class="Bool (strict)"("Value"=w343) -> ()  [unwired: 2 in, 2 out]
          }
          event User Event; "Tests List": Value Change {
            n156 = event-data() -> ()  [unwired: 1 in, 3 out]
            n157 = List Folder(path=w349, pattern="*.test") -> (path out=w350:path, filenames=w348:string[])  [unwired: 2 in, 2 out]
            n158 = property on="Tests List" class="LstBox (strict)"("Item Names"=w348) -> ()  [unwired: 2 in, 2 out]
            n159 = Array Size(array=w348) -> (size(s)=w355:i32)
            n160 = Not Equal To 0?(x=w355) -> (x != 0?=w354:bool)
            n161 = case shown="True" w354 {
              tunnel: w348 -> [_ w369]
              tunnel: w350 -> [_ w367]
              tunnel: w353 -> [w356 w359]
              tunnel: [w356 w358] -> w352
              frame False {
              }
              frame True {
                n162 = property on="Tests List" class="LstBox (strict)"() -> ("Value"=w357:i32)  [unwired: 2 in, 2 out]
                n163 = Index Array(array=w369, index=w357) -> (element=w368:string)
                n164 = Build Path(base path=w367, name or relative path=w368) -> (appended path=w366:path)
                n165 = call <vilib>:"Open_Create_Replace File.vi"("file path"=w366) -> ("error out"=w364:errorcluster, "file size (bytes)"=w363:i32, "refnum"=w365:refnum<file>)  [unwired: 7 in, 1 out]
                n166 = Read from Binary File(8:w364, 10:w363, 11:w365) -> (0:w361:errorcluster, 2:w360:string, 3:w362:refnum<file>)  [unwired: 3 in, 1 out]
                n167 = call "FindScriptPorts.vi"("Input FOR VOC"=w359, "Test"=w360) -> ("Result Input FOR VOC"=w358:u8[])
                "Result Input FOR VOC" <- w358
                n168 = Close File(refnum=w362, error in=w361) -> ()  [unwired: 2 out]
                n169 = property on="TEST" class="Str"(error in=w361, "Value"=w360) -> ()  [unwired: 1 in, 2 out]
              }
            }
          }
          event "Set new value\n(ALG ports)": Mouse Down {
            n170 = event-data() -> ()  [unwired: 1 in, 8 out]
            n171 = property on="ALG Input Ports" class="MCListbox (strict)"() -> ("Value"=w373:i32)  [unwired: 2 in, 2 out]
            n172 = property on="New value\n(ALG ports)" class="DigNum (strict)"() -> ("Value"=w372:i8)  [unwired: 2 in, 2 out]
            n173 = control-ref of="ALG Input Ports"() -> (w371:refnum<vi>)
            n174 = call "GUIUpdater.vi"("value"=w372, "Color"=u32 13260, "line"=w373, "MCListbox Refnum"=w371) -> ()
            n175 = Replace Array Subset(array=w375, new element=w372, index=w373) -> (w374:i32[])
            "output array 2" <- w374
          }
          event "Set new value (VOC ports)": Mouse Down {
            n176 = event-data() -> ()  [unwired: 1 in, 8 out]
            n177 = property on="VOC Input Ports" class="MCListbox (strict)"() -> ("Value"=w379:i32)  [unwired: 2 in, 2 out]
            n178 = property on="New value (VOC ports)" class="DigNum (strict)"() -> ("Value"=w385:i8)  [unwired: 2 in, 2 out]
            n179 = control-ref of="VOC Input Ports"() -> (w384:refnum<vi>)
            n180 = call "GUIUpdater.vi"("value"=w385, "Color"=u32 39219, "line"=w379, "MCListbox Refnum"=w384) -> ()
            n181 = Replace Array Subset(array=w383, new element=w385, index=w379) -> (w381:i32[])
            "output array 3" <- w381
          }
          event "Controlable\n(ALG ports)": Value Change {
            n182 = event-data() -> ("NewVal"=w389:bool)  [unwired: 1 in, 5 out]
            n183 = Not(x=w389) -> (.not. x?=w388:bool)
            n184 = Boolean To (0,1)(Boolean=w388) -> (0, 1=w392:i16)
            n185 = local read "ALG Port and states"() -> (w397:string[][])
            n186 = Multiply(x=w392, y=i16 2) -> (x*y=w390:i16)
            n187 = property on="ALG Input Ports" class="MCListbox (strict)"() -> ("Value"=w395:i32)  [unwired: 2 in, 2 out]
            n188 = property on="Set new value\n(ALG ports)" class="Bool (strict)"("Disabled"=w390) -> ()  [unwired: 2 in, 2 out]
            n189 = case shown="True" w389 {
              tunnel: w395 -> [w402 w409]
              tunnel: w397 -> [w403 w411]
              tunnel: [w404 w407] -> w396
              frame False {
                n190 = Replace Array Subset(array=w403, new element="НЕУПР", index (row)=w402, index (col)=1 ("disabled index (col)")) -> (w404:string[][])
              }
              frame True {
                n191 = Replace Array Subset(array=w411, new element="УПР", index (row)=w409, index (col)=1 ("disabled index (col)")) -> (w407:string[][])
              }
            }
            n192 = local read "ALG INPUT PORT states"() -> (w394:bool[])
            n193 = Replace Array Subset(array=w394, new element=w389, index=w395) -> (w393:bool[])
            n194 = local write "ALG Port and states"(w396) -> ()
            n195 = property on="ALG Input Ports" class="MCListbox (strict)"("Item Names"=w396) -> ()  [unwired: 2 in, 2 out]
            n196 = local write "ALG INPUT PORT states"(w393) -> ()
          }
          event "Controlable (VOC ports)": Value Change {
            n197 = event-data() -> ("NewVal"=w414:bool)  [unwired: 1 in, 5 out]
            n198 = Not(x=w414) -> (.not. x?=w413:bool)
            n199 = Boolean To (0,1)(Boolean=w413) -> (0, 1=w417:i16)
            n200 = property on="VOC Input Ports" class="MCListbox (strict)"() -> ("Value"=w412:i32)  [unwired: 2 in, 2 out]
            n201 = local read "VOC Port and states"() -> (w421:string[][])
            n202 = Multiply(x=w417, y=i16 2) -> (x*y=w415:i16)
            n203 = property on="Set new value (VOC ports)" class="Bool (strict)"("Disabled"=w415) -> ()  [unwired: 2 in, 2 out]
            n204 = case shown="True" w414 {
              tunnel: w412 -> [w426 w433]
              tunnel: w421 -> [w427 w435]
              tunnel: [w428 w431] -> w420
              frame False {
                n205 = Replace Array Subset(array=w427, new element="НЕУПР", index (row)=w426, index (col)=1 ("disabled index (col)")) -> (w428:string[][])
              }
              frame True {
                n206 = Replace Array Subset(array=w435, new element="УПР", index (row)=w433, index (col)=1 ("disabled index (col)")) -> (w431:string[][])
              }
            }
            n207 = local read "VOC INPUT PORT states"() -> (w419:bool[])
            n208 = Replace Array Subset(array=w419, new element=w414, index=w412) -> (w418:bool[])
            n209 = local write "VOC Port and states"(w420) -> ()
            n210 = property on="VOC Input Ports" class="MCListbox (strict)"("Item Names"=w420) -> ()  [unwired: 2 in, 2 out]
            n211 = local write "VOC INPUT PORT states"(w418) -> ()
          }
          event "Save changes in current test": Mouse Down {
            w443 = 0 ("pos offset (0)")
            n212 = event-data() -> ()  [unwired: 1 in, 8 out]
            n213 = property on="TEST" class="Str"() -> ("Value"=w440:string)  [unwired: 2 in, 2 out]
            n214 = property on="Tests List" class="LstBox (strict)"() -> ("Value"=w445:i32)  [unwired: 2 in, 2 out]
            n215 = property on="Tests List" class="LstBox (strict)"() -> ("Item Names"=w448:string[])  [unwired: 2 in, 2 out]
            n216 = Index Array(array=w448, index=w445) -> (element=w455:string)
            n217 = Build Path(base path=w449, name or relative path=w455) -> (appended path=w454:path)
            n218 = call <vilib>:"Open_Create_Replace File.vi"("function (open:0)"=T2."open", "file path"=w454) -> ("error out"=w441:errorcluster, "refnum"=w442:refnum<file>)  [unwired: 6 in, 2 out]
            n219 = call "FindScriptPorts.vi"("Input FOR VOC"=w451, "Test"=w440) -> ("Result Input FOR VOC"=w450:u8[])
            n220 = Set File Position(offset (in bytes) (0)=w443, refnum=w442, from (0:start)=w443, error in=w441) -> (refnum out=w438:refnum<file>, error out=w437:errorcluster)
            n221 = Write to Binary File(file (use dialog)=w438, data=w440, error in=w437, 5:FALSE ("prepend array or string size? (T)")) -> (refnum out=w453:refnum<file>, error out=w452:errorcluster)  [unwired: 2 in, 1 out]
            n222 = Close File(refnum=w453, error in=w452) -> ()  [unwired: 2 out]
          }
          event "ALG Param type": Value Change {
            n223 = event-data() -> ()  [unwired: 1 in, 6 out]
            n224 = property on="ALG Param type" class="CmbBox"() -> ("Value"=w461:string)  [unwired: 2 in, 2 out]
            n225 = property on="ALG Last Interation MSG" class="MCListbox (strict)"() -> ("Value"=w457:i32)  [unwired: 2 in, 2 out]
            n226 = Index Array(array=w460, index=w457) -> (element=w464:string)
            n227 = case shown="\"ПЛАВ\"" w461 {
              tunnel: w464 -> [w468 w473]
              tunnel: [w468 w471] -> w463
              frame "False", Default {
              }
              frame "ПЛАВ" {
                n228 = Decimal String To Number(string=w473) -> (number=w475:i32)  [unwired: 2 in, 1 out]
                n229 = Type Cast(type=sgl 0.0, x=w475) -> (*(type *) &x=w472:sgl)
                n230 = Number To Exponential String(number=w472, precision (6)=i16 3, 3:i16 10 ("width (-)")) -> (E-format string=w471:string)  [unwired: 1 in]
              }
            }
            n231 = property on="ALG Last Interation MSG" class="MCListbox (strict)"() -> ("Item Names"=w459:string[][])  [unwired: 2 in, 2 out]
            n232 = Replace Array Subset(array=w459, new element=w463, index (row)=w457, index (col)=1 ("disabled index (col)")) -> (w458:string[][])
            n233 = property on="ALG Last Interation MSG" class="MCListbox (strict)"("Item Names"=w458) -> ()  [unwired: 2 in, 2 out]
          }
          event "VOC Param type": Value Change {
            # "VOC output msg PARAM CASHE"
            n234 = event-data() -> ()  [unwired: 1 in, 6 out]
            n235 = property on="VOC Last Interation MSG" class="MCListbox (strict)"() -> ("Value"=w483:i32)  [unwired: 2 in, 2 out]
            n236 = property on="VOC Param type" class="CmbBox"() -> ("Value"=w485:string)  [unwired: 2 in, 2 out]
            n237 = Index Array(array=w486, index=w483) -> (element=w487:string)
            n238 = case shown="\"ПЛАВ\"" w485 {
              tunnel: w487 -> [w488 w493]
              tunnel: [w488 w491] -> w482
              frame "False", Default {
              }
              frame "ПЛАВ" {
                n239 = Decimal String To Number(string=w493) -> (number=w495:i32)  [unwired: 2 in, 1 out]
                n240 = Type Cast(type=sgl 0.0, x=w495) -> (*(type *) &x=w492:sgl)
                n241 = Number To Exponential String(number=w492, precision (6)=i16 3, 3:i16 10 ("width (-)")) -> (E-format string=w491:string)  [unwired: 1 in]
              }
            }
            n242 = property on="VOC Last Interation MSG" class="MCListbox (strict)"() -> ("Item Names"=w481:string[][])  [unwired: 2 in, 2 out]
            n243 = Replace Array Subset(array=w481, new element=w482, index (row)=w483, index (col)=1 ("disabled index (col)")) -> (w480:string[][])
            n244 = property on="VOC Last Interation MSG" class="MCListbox (strict)"("Item Names"=w480) -> ()  [unwired: 2 in, 2 out]
          }
          event "Save as new test": Mouse Down {
            n245 = event-data() -> ()  [unwired: 1 in, 8 out]
            n246 = call "Save new test"() -> ("Test name"=w504:string, "OK"=w503:bool)  [unwired: 17 in, 1 out]
            n247 = property on="TEST" class="Str"() -> ("Value"=w497:string)  [unwired: 2 in, 2 out]
            n248 = case shown="True" w503 {
              tunnel: w500 -> [_ w511]
              tunnel: w504 -> [_ w518]
              tunnel: w497 -> [_ w509]
              tunnel: w502 -> [w505 w508]
              tunnel: [w505 w507] -> w501
              frame False {
              }
              frame True {
                n249 = Concatenate Strings(w518, ".test" ("string")) -> (w512:string)
                n250 = Build Path(base path=w511, name or relative path=w512) -> (appended path=w513:path)
                n251 = call "FindScriptPorts.vi"("Input FOR VOC"=w508, "Test"=w509) -> ("Result Input FOR VOC"=w507:u8[])
                n252 = call <vilib>:"Open_Create_Replace File.vi"("function (open:0)"=T2."open or create", "file path"=w513) -> ("error out"=w517:errorcluster, "refnum"=w514:refnum<file>)  [unwired: 6 in, 2 out]
                n253 = Write to Binary File(file (use dialog)=w514, data=w509, error in=w517, 5:FALSE ("prepend array or string size? (T)")) -> (refnum out=w515:refnum<file>, error out=w516:errorcluster)  [unwired: 2 in, 1 out]
                n254 = Close File(refnum=w515, error in=w516) -> ()  [unwired: 2 out]
              }
            }
          }
        }
        n255 = property on="run" class="Bool (strict)"() -> ("Value"=w241:bool)  [unwired: 2 in, 2 out]
        n256 = case shown="True" w241 {
          tunnel: w259 -> [w535 w584]
          tunnel: w258 -> [w529 w583]
          tunnel: w219 -> [w534 w582]
          tunnel: w257 -> [w531 w581]
          tunnel: w256 -> [w532 w580]
          tunnel: w255 -> [w533 w579]
          tunnel: w254 -> [w530 w578]
          tunnel: w253 -> [w528 w577]
          tunnel: w229 -> [_ w576]
          tunnel: w228 -> [_ w555]
          tunnel: w252 -> [_ w575]
          tunnel: w251 -> [_ w574]
          tunnel: w250 -> [_ w573]
          tunnel: w249 -> [_ w572]
          tunnel: [w535 w571] -> w248
          tunnel: [w534 w570] -> w247
          tunnel: [w533 w569] -> w246
          tunnel: [w532 w568] -> w226
          tunnel: [w531 w567] -> w227
          tunnel: [w530 w566] -> w244
          tunnel: [w528 w565] -> w243
          tunnel: [w529 w552] -> w242
          tunnel: w240 -> [w527 w539]
          tunnel: [w527 w538] -> w239
          tunnel: w238 -> [_ w563]
          tunnel: w237 -> [_ w562]
          tunnel: w236 -> [_ w561]
          tunnel: w225 -> [_ w560]
          tunnel: w235 -> [w526 w559]
          tunnel: [w526 w558] -> w234
          tunnel: w233 -> [w525 w557]
          tunnel: [w525 w556] -> w232
          tunnel: w231 -> [w524 w537]
          tunnel: [w524 w536] -> w230
          tunnel: w223 -> [w523 w541]
          tunnel: [w523 w554] -> w224
          tunnel: w222 -> [w522 w543]
          tunnel: [w522 w553] -> w221
          frame False {
          }
          frame True {
            n257 = flat-sequence {
              tunnel: w584 -> [w625]
              tunnel: w583 -> [w626]
              tunnel: w582 -> [w602]
              tunnel: w581 -> [w624]
              tunnel: w580 -> [w623]
              tunnel: w579 -> [w622]
              tunnel: w578 -> [w619]
              tunnel: w577 -> [w621]
              tunnel: w576 -> [w620]
              tunnel: w555 -> [w618]
              tunnel: [w617] -> w551
              tunnel: [w616] -> w549
              tunnel: [w588] -> w571
              tunnel: [w595] -> w570
              tunnel: [w614] -> w569
              tunnel: [w601] -> w568
              tunnel: [w615] -> w567
              tunnel: [w600] -> w566
              tunnel: [w613] -> w565
              tunnel: [w612] -> w547
              tunnel: [w611] -> w564
              tunnel: w563 -> [w610]
              tunnel: w562 -> [w599]
              tunnel: w561 -> [w609]
              tunnel: w560 -> [w608]
              tunnel: w559 -> [w607]
              tunnel: [w606] -> w558
              tunnel: w557 -> [w605]
              tunnel: [w604] -> w556
              tunnel: [w603] -> w545
              tunnel: w551 -> [w682]
              tunnel: [w682] -> w550
              tunnel: w549 -> [w681]
              tunnel: [w681] -> w548
              tunnel: w547 -> [w680]
              tunnel: [w680] -> w546
              tunnel: w545 -> [w679]
              tunnel: [w679] -> w544
              tunnel: w543 -> [w678]
              tunnel: [w678] -> w542
              tunnel: w541 -> [w677]
              tunnel: [w677] -> w540
              tunnel: w539 -> [w674]
              tunnel: [w673] -> w538
              tunnel: w537 -> [w666]
              tunnel: [w665] -> w536
              tunnel: [w707] -> w552
              tunnel: w550 -> [w705]
              tunnel: w575 -> [w706]
              tunnel: w574 -> [w711]
              tunnel: w573 -> [w710]
              tunnel: w572 -> [w709]
              tunnel: w548 -> [w708]
              tunnel: w546 -> [w707]
              tunnel: w564 -> [w704]
              tunnel: w544 -> [w698]
              tunnel: [w702] -> w554
              tunnel: [w695] -> w553
              tunnel: w542 -> [w694]
              tunnel: w540 -> [w693]
              frame #0 {
                n258 = local read "Mode"() -> (w628:bool)
                n259 = case shown="False" w628 {
                  tunnel: [w637 1] -> w627
                  frame False {
                    # "STEP MODE"
                    n260 = local read "STEP SIZE"() -> (w637:i32)
                    n261 = property on="stop 2" class="Bool (strict)"("Value"=TRUE ("stop")) -> ()  [unwired: 2 in, 2 out]
                    n262 = property on="run" class="Bool (strict)"("Value"=FALSE ("run")) -> ()  [unwired: 2 in, 2 out]
                  }
                  frame True {
                    # "CONTINUOUS MODE"
                  }
                }
                n263 = for {
                  N: w627 -> [_]
                  shift-right: [w645] -> w591
                  shift-left: w625 -> [w664]
                  shift-right: [w646] -> w594
                  shift-left: w602 -> [w663]
                  shift-right: [w648] -> w615
                  shift-left: w624 -> [w652]
                  shift-right: [w658] -> w601
                  shift-left: w623 -> [w659]
                  shift-right: [w644] -> w600
                  shift-left: w619 -> [w651]
                  shift-right: [w649] -> w614
                  shift-left: w622 -> [w650]
                  shift-right: [w656] -> w612
                  shift-left: w626 -> [w661]
                  tunnel: w621 -> [w660]
                  shift-right: [w647] -> w617
                  shift-left: w620 -> [w662]
                  shift-right: [w642] -> w616
                  shift-left: w618 -> [w643]
                  tunnel: [w657] -> w613
                  tunnel: [w655] -> w611
                  tunnel: [w641] -> w603
                  n264 = call "VOC.vi"("input VOC ports"=w664, "voc states array"=w659, "output VOC ports"=w663, "Input VOC msg Array"=w661, "output VOC msg array"=w660, "VOC output msg CASHE"=w662) -> ("Filled voc states array"=w658:cluster{u32, u8}[], "Modified input VOC ports"=w654:u8[], "Modified output VOC ports"=w653:u8[], "Clear Input VOC msg Array"=w656:cluster{i32, "Value":string, i32}[], "clear output VOC array"=w657:cluster{i32, "Value":string, i32}[], "Curr step output MSG counter"=w655:i32, "Filled VOC output msg CASHE"=w647:cluster{i32, "Value":string, i32}[])  [unwired: 3 in]
                  n265 = call "CA.vi"("init input ports"=w653, "Alg states"=w650, "output"=w654, "input ALG msg array"=w652, "Output ALG msg array"=w651, "VOC output msg CASHE"=w647, "ALG output msg CASHE"=w643) -> ("Output Alg states"=w649:cluster{u32, u8}[], "input ports"=w646:u8[], "modified output ports"=w645:i8[], "Clear ALG input array"=w648:cluster{i32, "Value":string, i32}[], "Clear ALG output array"=w644:cluster{i32, "Value":string, i32}[], "Curr step msg counter"=w641:i32, "Modified ALG output msg CASHE"=w642:cluster{i32, "Value":string, i32}[])  [unwired: 2 in]
                }
                "Alg Input" <- w594
                n266 = local read "Init  VOC INPUT"() -> (w590:u8[])
                n267 = local read "VOC INPUT PORT states"() -> (w589:bool[])
                n268 = local read "ALG INPUT PORT states"() -> (w597:bool[])
                n269 = local read "Init ALG input"() -> (w593:u8[])
                n270 = call "PSConverter.vi"("Current States 2"=w607, "PROC"=w610, "STATES"=w599, "Input claster"=w614) -> ("Current States"=w606:string[][])
                n271 = property on="Alg States" class="Tbl (strict)"("Value"=w606) -> ()  [unwired: 2 in, 2 out]
                n272 = call "PSConverter.vi"("Current States 2"=w605, "PROC"=w609, "STATES"=w608, "Input claster"=w601) -> ("Current States"=w604:string[][])
                n273 = call "PortsArrayHandler.vi"("Input"=w591, "Init Input"=w590, "INPUT PORT states"=w589) -> ("Rezult Input Ports"=w588:i32[], "boolean Ports Array"=→"Output Alg Ports":bool[])
                n274 = call "PortsArrayHandler.vi"("Input"=w594, "Init Input"=w593, "INPUT PORT states"=w597) -> ("Rezult Input Ports"=w595:i32[], "boolean Ports Array"=→"Input Alg Ports":bool[])
                n275 = property on="VOC States" class="Tbl (strict)"("Value"=w604) -> ()  [unwired: 2 in, 2 out]
                n276 = control-ref of="VOC Input Ports"() -> (w587:refnum<vi>)
                n277 = for {
                  tunnel: w588 -> [w631] mode=indexing
                  tunnel: w587 -> [w630]
                  tunnel: u32 3394560 -> [w629]
                  i -> [w632]
                  n278 = call "GUIUpdater.vi"("value"=w631, "Color"=w629, "line"=w632, "MCListbox Refnum"=w630) -> ()
                }
                n279 = control-ref of="ALG Input Ports"() -> (w598:refnum<vi>)
                n280 = for {
                  tunnel: w595 -> [w635] mode=indexing
                  tunnel: w598 -> [w634]
                  tunnel: u32 13260 -> [w633]
                  i -> [w636]
                  n281 = call "GUIUpdater.vi"("value"=w635, "Color"=w633, "line"=w636, "MCListbox Refnum"=w634) -> ()
                }
                "Init  VOC INPUT" <- w625
                "Init ALG input" <- w602
              }
              frame #1 {
                n282 = local read "Curr step VOC MSG counter"() -> (w676:i32)
                n283 = local read "Curr step ALG msg counter"() -> (w667:i32)
                n284 = property on="VOC Last Interation MSG" class="MCListbox (strict)"() -> ("Item Names"=w669:string[][])  [unwired: 2 in, 2 out]
                n285 = property on="Output Alg Msg" class="Tbl (strict)"() -> ("Value"=w668:string[][])  [unwired: 2 in, 2 out]
                n286 = property on="ALG Last Interation MSG" class="MCListbox (strict)"() -> ("Item Names"=w671:string[][])  [unwired: 2 in, 2 out]
                n287 = property on="Output VOC Msg LOG" class="Tbl (strict)"() -> ("Value"=w670:string[][])  [unwired: 2 in, 2 out]
                n288 = call "MsgParser.vi"("Result Output Msg Table"=w670, "Output VOC Msg LOG"=w669, "MSG Counter"=w674, "current msg num"=w676) -> ("Result Counter"=w673:i32, "Output Alg Msg"=→"Output VOC Msg LOG":string[][])
                n289 = call "MsgParser.vi"("Result Output Msg Table"=w668, "Output VOC Msg LOG"=w671, "MSG Counter"=w666, "current msg num"=w667) -> ("Result Counter"=w665:i32, "Output Alg Msg"=→"Output Alg Msg":string[][])
              }
              frame #2 {
                # "Output VOC Msg"
                n290 = local read "Output VOC Msg Last Iter"() -> (w692:string[][])
                n291 = local read "Output ALG Msg Last Iter"() -> (w684:string[][])
                n292 = Array Size(array=w694) -> (size(s)=w697:i32)
                n293 = for {
                  N: w697 -> [_]
                  shift-right: [w729] -> w696
                  shift-left: w694 -> [w731]
                  i -> [w730]
                  n294 = Replace Array Subset(array=w731, new element="*" ("new element/subarray"), index=w730) -> (w729:string[])
                }
                n295 = Array Size(array=w692) -> (size(s)=w691:i32[])
                n296 = Array Size(array=w684) -> (size(s)=w687:i32[])
                n297 = Index Array(array=w691, index=0) -> (element=w689:i32)
                n298 = Index Array(array=w687, index=0) -> (element=w685:i32)
                n299 = Array Size(array=w693) -> (size(s)=w701:i32)
                n300 = for {
                  N: w689 -> [_]
                  shift-right: [w721] -> w688
                  shift-left: w692 -> [w728]
                  i -> [w722]
                  n301 = Replace Array Subset(array=w728, new element="" ("new element/subarray"), index (row)=w722, index (col)=0 ("disabled index (col)")) -> (w723:string[][])
                  n302 = Replace Array Subset(array=w723, new element="" ("new element/subarray"), index (row)=w722, index (col)=1 ("disabled index (col)")) -> (w721:string[][])
                }
                n303 = for {
                  N: w685 -> [_]
                  shift-right: [w713] -> w683
                  shift-left: w684 -> [w720]
                  i -> [w714]
                  n304 = Replace Array Subset(array=w720, new element="" ("new element/subarray"), index (row)=w714, index (col)=0 ("disabled index (col)")) -> (w715:string[][])
                  n305 = Replace Array Subset(array=w715, new element="" ("new element/subarray"), index (row)=w714, index (col)=1 ("disabled index (col)")) -> (w713:string[][])
                }
                n306 = for {
                  N: w701 -> [_]
                  shift-right: [w733] -> w699
                  shift-left: w693 -> [w735]
                  i -> [w734]
                  n307 = Replace Array Subset(array=w735, new element="*" ("new element/subarray"), index=w734) -> (w733:string[])
                }
                n308 = call "LastStepMsgParser.vi"("Params array"=w696, "Output Msg Table"=w688, "Out MSG Codes"=w711, "output msg array"=w705, "Out MSG Names"=w706, "current msg num"=w704) -> ("Params"=w695:string[], "code"=→"voc code":i32[], "Output Alg Msg"=w703:string[][])  [unwired: 2 in]
                n309 = property on="VOC Last Interation MSG" class="MCListbox (strict)"("Item Names"=w703) -> ()  [unwired: 2 in, 2 out]
                n310 = call "LastStepMsgParser.vi"("Params array"=w699, "Output Msg Table"=w683, "Out MSG Codes"=w710, "output msg array"=w708, "Out MSG Names"=w709, "current msg num"=w698) -> ("Params"=w702:string[], "Output Alg Msg"=w700:string[][])  [unwired: 2 in, 1 out]
                "Params" <- w702
                n311 = property on="ALG Last Interation MSG" class="MCListbox (strict)"("Item Names"=w700) -> ()  [unwired: 2 in, 2 out]
                "Curr step VOC MSG counter" <- w704
                "Curr step ALG msg counter" <- w698
              }
            }
          }
        }
        n312 = local read "Mode"() -> (w268:bool)
        n313 = case shown="False" w268 {
          tunnel: [u32 0 ("millisecond multiple") u32 0 ("millisecond multiple")] -> w267
          frame False {
          }
          frame True {
            # "CONTINUOUS MODE"
          }
        }
        n314 = Wait Until Next ms Multiple(millisecond multiple=w267) -> ()  [unwired: 1 out]
      }
    }
  }
